vi "AeroQuadConfigurator.vi"() -> ()   [LabVIEW 2010]
uses:
  <vilib>/Utility/config.llb/Config Data RefNum.ctl
  <vilib>/Utility/miscctls.llb/LVRowAndColumnTypeDef.ctl
  <vilib>/Utility/miscctls.llb/LVRowAndColumnUnsignedTypeDef.ctl
  <vilib>/Utility/config.llb/Read Key (Double).vi
  <vilib>/Utility/config.llb/Read Key (String).vi
  <vilib>/Utility/config.llb/Read Key (I32).vi
  <vilib>/Utility/config.llb/Write Key (I32).vi
  <vilib>/Utility/config.llb/Write Key (String).vi
  <vilib>/Platform/browser.llb/Open URL in Default Browser (string).vi
  <vilib>/Instr/_visa.llb/VISA Configure Serial Port (Instr).vi
  <vilib>/Utility/config.llb/NI_LVConfig.lvlib
panel:
  out "LargeStatus":string
  in  "Load SubPanel":i32(ring) caption="Information Display" items=["Initial Setup", "3-D View", "Vehicle Status", "Map Tracker", "Motor Commands", "Serial Monitor", "Vehicle Attitude", "Sensor Data", "Transmitter Data"]
  in  "Parameter Type":i32(ring) caption="Configuration" items=["Rate Mode", "Attitude Mode", "Yaw Configuration", "Altitude Hold", "Miscellaneous Configuration", "Transmitter Smoothing", "Battery Monitor", "Camera Stabilization"]
  in  "Parameter Check":string[][](table)
  in  "Upload":bool
  out "Sensors":string[][](table)
  out "Status":string="AeroQuad Configurator"
  in  "*Com Port":refnum<visa-resource-name> caption="Com Port"
  in  "*Baud Rate":string(combo)="115200" caption="Baud Rate"
  in  "*Timeout (sec)":dbl=3.0 caption="Timeout (sec)"
  in  "Open Port":bool
  in  "Disconnect":bool
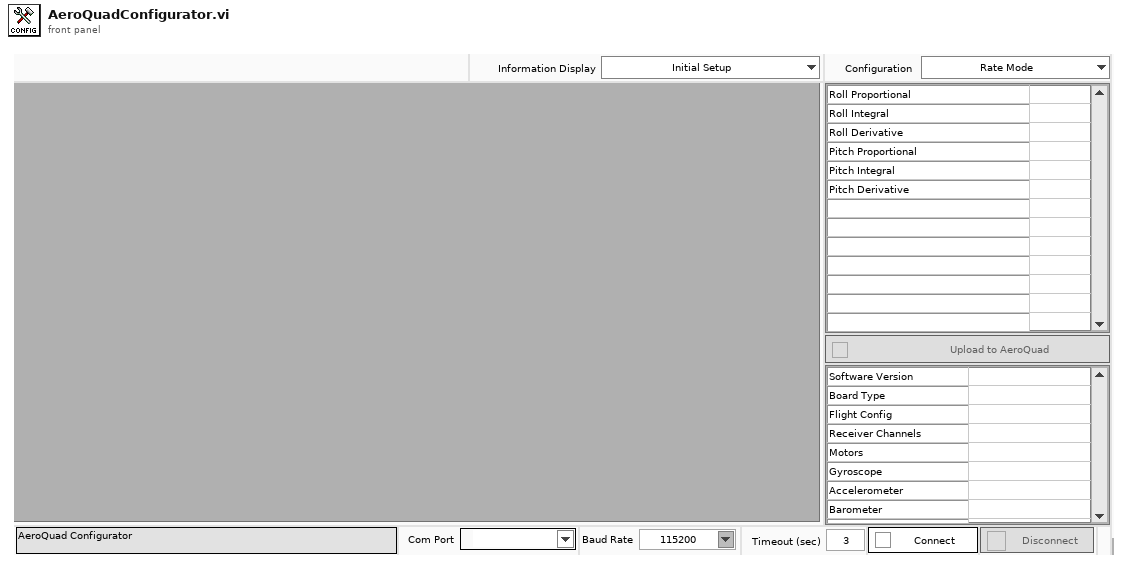
[diagram p1: front panel]
types:
  T1 = typedef "NI_LVConfig.lvlib/Config Data RefNum.ctl" = refnum<k1>
  T2 = cluster{"Error":errorcluster, "Data":dbl[], "COM Port":refnum<visa-resource-name>, "Data Type":enum16{"Serial", "Binary"}, "Connected":bool, "Parameters":string[][][], "WorkingPath":path, "ConfigRef":T1, "SubPanelName":string[], "ParameterName":string[], "Plots":string[][][], "SubPanelQueue":refnum<queue>, "SubPanel":refnum<vi>, "Debug":bool, "SubPanelType":string[], "Version":string, "StopTelem":string, "Config":string[][], "oldTelem":string, "previousValid":string, "oldCmd":string, "StartDelay":dbl, "ParamDesc":string[][], "IniPath":path, "SW":string}
  T3 = enum8{"Enabled", "Disabled", "Disabled and Grayed Out"}
  T4 = cluster{"Section":string, "Key":string, "Value":string}
  T5 = typedef "LVRowAndColumnTypeDef.ctl" = cluster{"Row":i32, "Column":i32}
  T6 = typedef "LVRowAndColumnUnsignedTypeDef.ctl" = cluster{"Row":u32, "Column":u32}
  T7 = enum32{"invalid app kind", "Development System", "Run Time System", "Student Edition", "Embedded LabVIEW", "Evaluation", "Custom"}
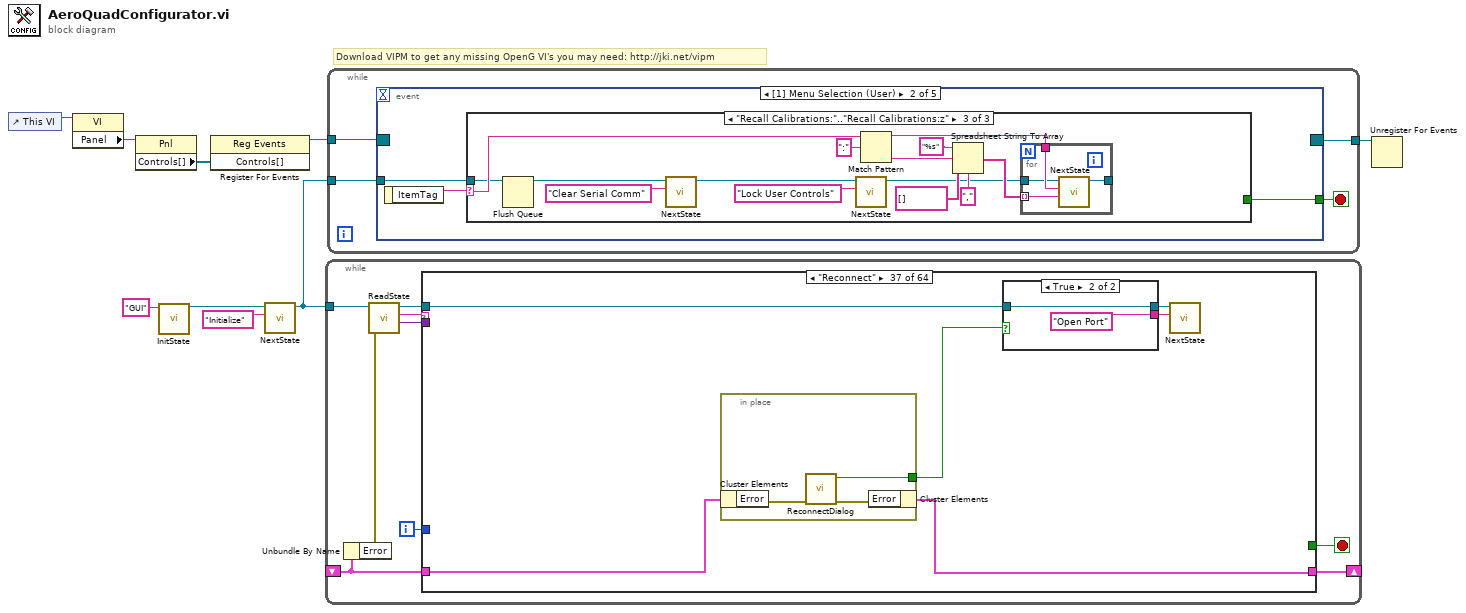
[diagram p0: block diagram]
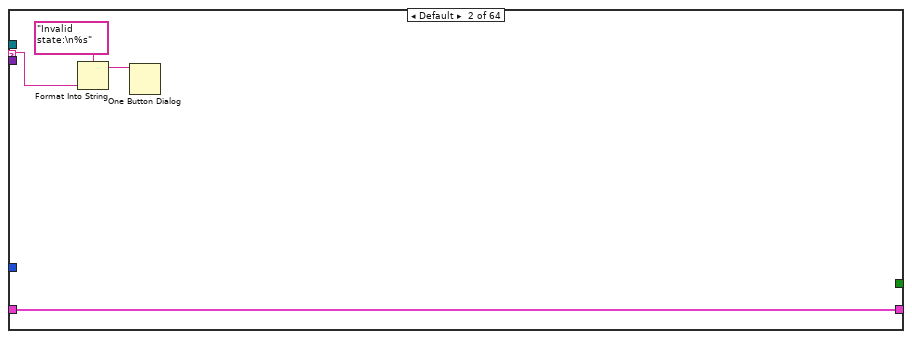
[diagram p3: hidden frame]
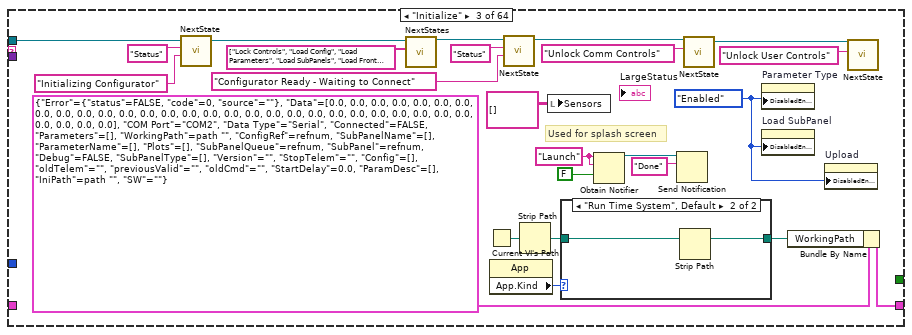
[diagram p4: hidden frame]
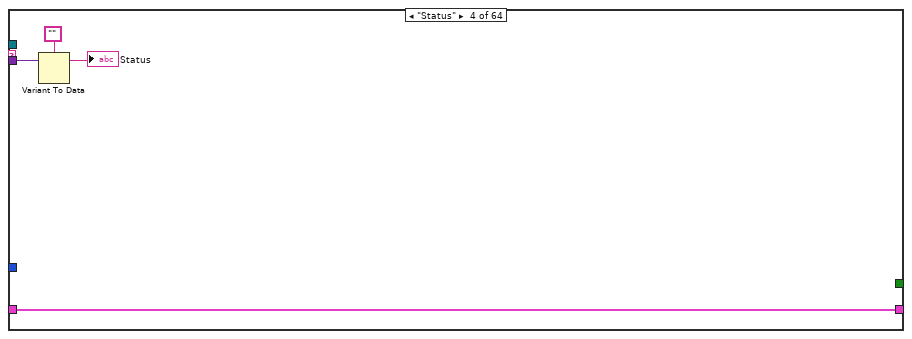
[diagram p6: hidden frame]
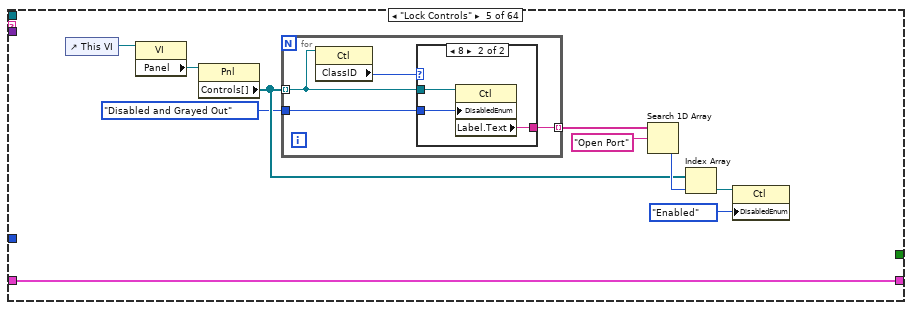
[diagram p7: hidden frame]
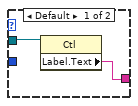
[diagram p8: hidden frame]
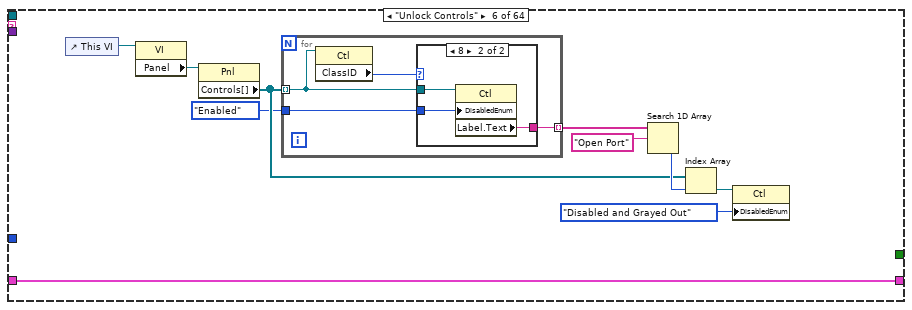
[diagram p9: hidden frame]
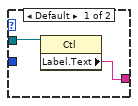
[diagram p10: hidden frame]
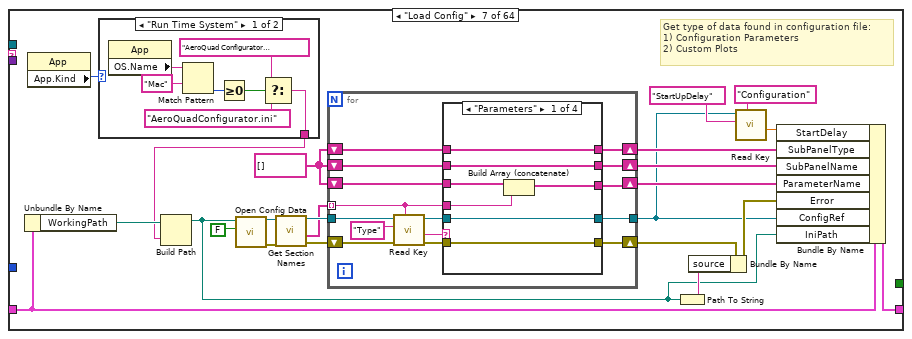
[diagram p11: hidden frame]
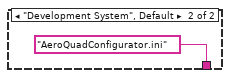
[diagram p12: hidden frame]
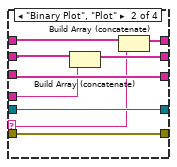
[diagram p13: hidden frame]
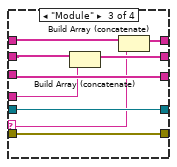
[diagram p14: hidden frame]
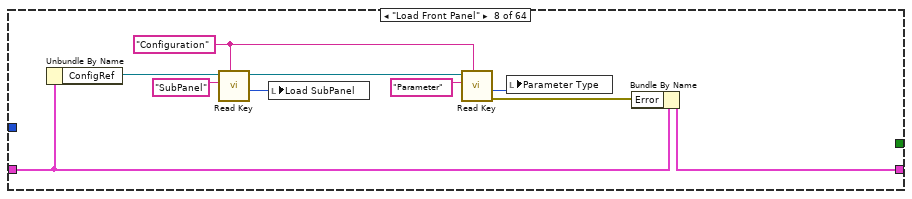
[diagram p16: hidden frame]
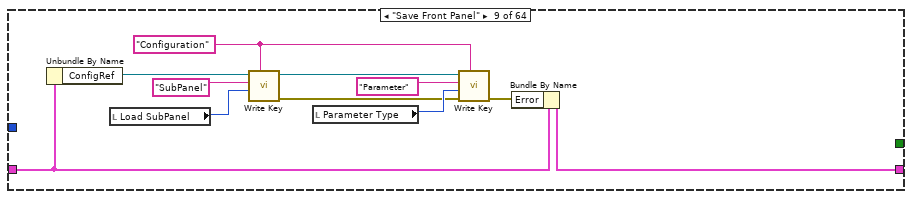
[diagram p17: hidden frame]
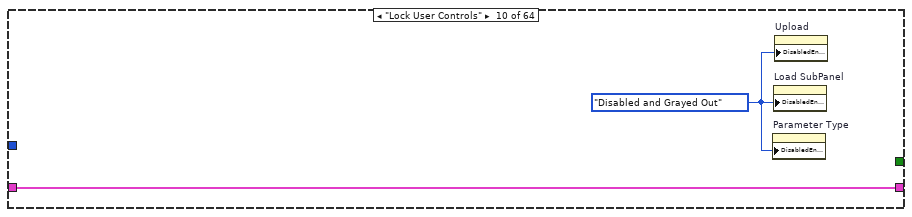
[diagram p18: hidden frame]
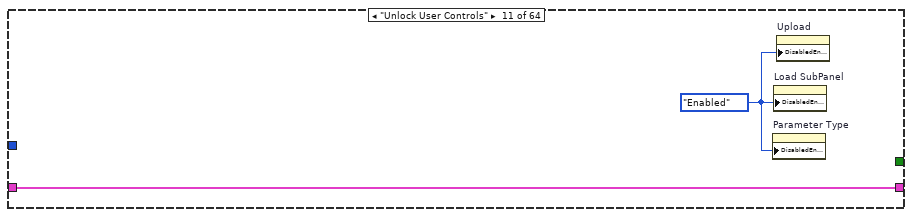
[diagram p19: hidden frame]
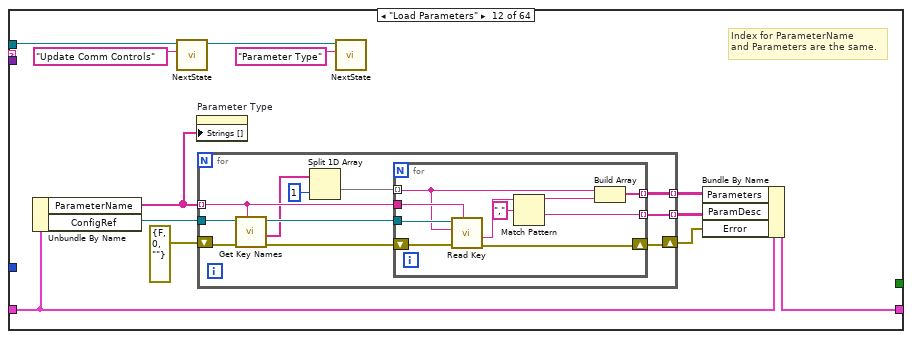
[diagram p20: hidden frame]
diagram:
  # "Download VIPM to get any missing OpenG VI's you may need: http://jki.net/vipm"
  n1 = control-ref of="This VI"() -> (w9:refnum<vi>)
  n2 = property class="VI"(reference=w9) -> ("Panel"=w8:refnum<vi>)  [unwired: 1 in, 2 out]
  n3 = property class="Pnl"(reference=w8) -> ("Controls[]"=w7:refnum<vi>[])  [unwired: 1 in, 2 out]
  n4 = call "InitState.vi"("Name"="GUI") -> ("Queue Out"=w2:refnum<queue>)  [unwired: 8 in, 1 out]
  n5 = register-events(w7) -> (reference out=w6:refnum<event-registration>)  [unwired: 2 in, 1 out]
  n6 = call "NextState.vi"("State"="Initialize", "Queue In"=w2) -> ("Queue Out"=w3:refnum<queue>)  [unwired: 8 in, 1 out]
  n7 = while {
    tunnel: w3 -> [w13]
    shift-right: [w18] -> _
    shift-left: _ -> [w15]
    i -> [w16]
    stop <- w17 stop-if-true
    n8 = Unbundle By Name(w15) -> ("Error"=w14:errorcluster)
    n9 = call "ReadState.vi"("Error In"=w14, "Queue In"=w13) -> ("Data"=w10:variant, "State"=w11:string, "Queue Out"=w12:refnum<queue>)  [unwired: 6 in, 1 out]
    n10 = case shown="\"Reconnect\"" w11 {
      tunnel: w10 -> [_ _ _ w51 _ _ _ _ _ _ _ _ _ w248 w263 _ _ _ w320 w326 _ _ _ _ _ _ _ _ _ w482 w486 _ _ _ w623 _ _ _ w689 _ _ _ _ _ _ _ w892 _ _ _ _ _ _ w993 _ _ _ w1117 w1132 _ _ w1241 w1253 w1321]
      selector: w11 -> [_ w22 _ _ _ _ _ _ _ _ _ _ _ _ w253 _ _ _ _ _ _ _ _ _ _ _ _ _ _ _ _ _ _ _ w619 _ _ _ _ _ _ _ _ _ _ _ _ _ _ _ _ _ _ _ _ _ _ _ _ _ _ w1240 w1252 _]
      tunnel: [w19 w23 w36 w52 w56 w75 w111 w171 w187 w191 w193 w204 w237 w250 w264 w282 w314 w317 w321 w327 w329 w339 w342 w377 w432 w433 w462 w474 w476 w481 w487 w506 w540 w596 w624 w640 w664 w684 w686 w695 w697 w711 w743 w758 w820 w881 w890 w905 w906 w910 w931 w948 w967 w995 w1044 w1050 w1052 w1120 w1180 w1186 w1223 w1236 w1250 w1327] -> w18
      tunnel: [_ _ _ _ _ _ _ _ _ _ _ _ _ _ _ _ _ _ _ _ _ TRUE _ _ _ _ _ _ _ _ _ _ _ _ _ _ _ _ _ _ _ _ _ _ _ _ _ _ _ _ _ _ _ _ _ _ _ _ _ _ _ _ _ _] -> w17
      tunnel: w15 -> [w19 w23 _ w52 w56 w75 w112 w172 w188 w191 w193 w205 w238 w251 w264 w283 w314 w317 w321 w327 w329 w339 w342 w378 w432 w434 w462 w474 w476 w481 w487 w492 w541 w597 w625 w641 w665 w685 w686 w695 w697 w711 w743 w759 w821 w881 w890 w905 w906 w911 w932 w949 w968 w996 w1044 w1050 w1053 w1120 w1180 w1186 w1223 w1237 w1250 w1327]
      tunnel: w16 -> [_ _ _ _ _ _ _ _ _ _ _ _ _ _ _ w284 _ _ _ _ _ _ _ _ _ _ _ _ _ _ _ _ _ _ _ _ _ _ _ _ _ _ _ _ _ _ _ _ _ _ _ _ _ _ _ _ _ _ _ _ _ _ _ _]
      tunnel: w12 -> [_ _ w47 _ _ _ _ _ _ _ _ w198 w228 _ w257 w280 _ w316 _ _ _ w340 _ w351 _ _ _ _ _ _ w483 w497 w543 w595 w620 _ w663 w681 _ _ _ _ _ _ _ w835 _ w894 _ w908 w929 _ w964 w990 w1038 _ w1054 w1115 w1145 _ _ _ w1247 w1326]
      frame "--- System ---" {
      }
      frame Default {
        n11 = Format Into String(format string="Invalid state:\n%s", w22) -> (resulting string=w20:string)  [unwired: 2 in, 1 out]
        n12 = One Button Dialog(message=w20) -> ()  [unwired: 1 in, 1 out]
      }
      frame "Initialize" {
        w27 = "Launch" ("name (unnamed)")
        w28 = T3."Enabled" ("Disabled")
        # "Used for splash screen"
        n13 = call "NextState.vi"("Data"="Initializing Configurator", "State"="Status", "Queue In"=w47) -> ("Queue Out"=w30:refnum<queue>)  [unwired: 7 in, 1 out]
        n14 = call "NextStates.vi"("States"=string[] ["Lock Controls", "Load Config", "Load Parameters", "Load SubPanels", "Load Front Panel"], "Queue In"=w30) -> ("Queue Out"=w29:refnum<queue>)  [unwired: 8 in, 1 out]
        n15 = Current VI's Path() -> (path=w39:path)
        n16 = property class="App"() -> ("App.Kind"=w41:T7)  [unwired: 2 in, 2 out]
        n17 = call "NextState.vi"("Data"="Configurator Ready - Waiting to Connect", "State"="Status", "Queue In"=w29) -> ("Queue Out"=w35:refnum<queue>)  [unwired: 7 in, 1 out]
        n18 = Strip Path(path=w39) -> (stripped path=w40:path)  [unwired: 1 out]
        n19 = local write "Sensors"(string[][] [] ("Sensors")) -> ()
        n20 = case shown="\"Run Time System\", Default" w41 {
          tunnel: w40 -> [w48 w50]
          tunnel: [w48 w49] -> w38
          frame "Development System" {
          }
          frame "Run Time System", Default {
            n21 = Strip Path(path=w50) -> (stripped path=w49:path)  [unwired: 1 out]
          }
        }
        n22 = Obtain Notifier(name (unnamed)=w27, notification data type=w27, create if not found? (T)=FALSE) -> (notifier out=w25:refnum<notifier>)  [unwired: 1 in, 2 out]
        n23 = Send Notification(notification="Done", notifier=w25) -> ()  [unwired: 1 in, 2 out]
        n24 = call "NextState.vi"("State"="Unlock Comm Controls", "Queue In"=w35) -> ("Queue Out"=w33:refnum<queue>)  [unwired: 8 in, 1 out]
        n25 = property on="Parameter Type" class="Ring (strict)"("DisabledEnum"=w28) -> ()  [unwired: 2 in, 2 out]
        n26 = property on="Load SubPanel" class="Ring (strict)"("DisabledEnum"=w28) -> ()  [unwired: 2 in, 2 out]
        n27 = Bundle By Name(cluster=T2 {"Error"={"status"=FALSE, "code"=0, "source"=""}, "Data"=[0.0, 0.0, 0.0, 0.0, 0.0, 0.0, 0.0, 0.0, 0.0, 0.0, 0.0, 0.0, 0.0, 0.0, 0.0, 0.0, 0.0, 0.0, 0.0, 0.0, 0.0, 0.0, 0.0, 0.0, 0.0, 0.0, 0.0, 0.0, 0.0, 0.0, 0.0, 0.0], "COM Port"="COM2", "Data Type"=enum."Serial", "Connected"=FALSE, "Parameters"=[], "WorkingPath"=path "", "ConfigRef"=refnum, "SubPanelName"=[], "ParameterName"=[], "Plots"=[], "SubPanelQueue"=refnum, "SubPanel"=refnum, "Debug"=FALSE, "SubPanelType"=[], "Version"="", "StopTelem"="", "Config"=[], "oldTelem"="", "previousValid"="", "oldCmd"="", "StartDelay"=0.0, "ParamDesc"=[], "IniPath"=path "", "SW"=""}, "WorkingPath"=w38) -> (w36:T2)
        n28 = property on="Upload" class="Bool"("DisabledEnum"=w28) -> ()  [unwired: 2 in, 2 out]
        n29 = call "NextState.vi"("State"="Unlock User Controls", "Queue In"=w33) -> ()  [unwired: 8 in, 2 out]
      }
      frame "Status" {
        n30 = Variant To Data(Variant=w51, type="") -> (data=→"Status":string)  [unwired: 1 in, 1 out]
      }
      frame "Lock Controls" {
        n31 = control-ref of="This VI"() -> (w63:refnum<vi>)
        n32 = property class="VI"(reference=w63) -> ("Panel"=w64:refnum<vi>)  [unwired: 1 in, 2 out]
        n33 = property class="Pnl"(reference=w64) -> ("Controls[]"=w59:refnum<vi>[])  [unwired: 1 in, 2 out]
        n34 = for {
          tunnel: w59 -> [w67] mode=indexing
          tunnel: [w68] -> w62 mode=indexing
          tunnel: T3."Disabled and Grayed Out" ("Disabled") -> [w65]
          n35 = property class="Ctl"(reference=w67) -> ("ClassID"=w66:u32)  [unwired: 1 in, 2 out]
          n36 = case shown="8" w66 {
            tunnel: [w69 w73] -> w68
            tunnel: w67 -> [w70 w72]
            tunnel: w65 -> [_ w71]
            frame Default {
              n37 = property class="Ctl"(reference=w70) -> ("Label.Text"=w69:string)  [unwired: 1 in, 2 out]
            }
            frame 8 {
              n38 = property class="Ctl"(reference=w72, "DisabledEnum"=w71) -> ("Label.Text"=w73:string)  [unwired: 1 in, 2 out]
            }
          }
        }
        n39 = Search 1D Array(1D array=w62, element="Open Port") -> (index of element=w60:i32)  [unwired: 1 in]
        n40 = Index Array(array=w59, index=w60) -> (element=w58:refnum<vi>)
        n41 = property class="Ctl"(reference=w58, "DisabledEnum"=T3."Enabled" ("Disabled")) -> ()  [unwired: 1 in, 2 out]
      }
      frame "Unlock Controls" {
        n42 = control-ref of="This VI"() -> (w82:refnum<vi>)
        n43 = property class="VI"(reference=w82) -> ("Panel"=w83:refnum<vi>)  [unwired: 1 in, 2 out]
        n44 = property class="Pnl"(reference=w83) -> ("Controls[]"=w78:refnum<vi>[])  [unwired: 1 in, 2 out]
        n45 = for {
          tunnel: w78 -> [w86] mode=indexing
          tunnel: [w87] -> w81 mode=indexing
          tunnel: T3."Enabled" ("Disabled") -> [w84]
          n46 = property class="Ctl"(reference=w86) -> ("ClassID"=w85:u32)  [unwired: 1 in, 2 out]
          n47 = case shown="8" w85 {
            tunnel: [w88 w92] -> w87
            tunnel: w86 -> [w89 w91]
            tunnel: w84 -> [_ w90]
            frame Default {
              n48 = property class="Ctl"(reference=w89) -> ("Label.Text"=w88:string)  [unwired: 1 in, 2 out]
            }
            frame 8 {
              n49 = property class="Ctl"(reference=w91, "DisabledEnum"=w90) -> ("Label.Text"=w92:string)  [unwired: 1 in, 2 out]
            }
          }
        }
        n50 = Search 1D Array(1D array=w81, element="Open Port") -> (index of element=w79:i32)  [unwired: 1 in]
        n51 = Index Array(array=w78, index=w79) -> (element=w77:refnum<vi>)
        n52 = property class="Ctl"(reference=w77, "DisabledEnum"=T3."Disabled and Grayed Out" ("Disabled")) -> ()  [unwired: 1 in, 2 out]
      }
      frame "Load Config" {
        w98 = string[] []
        # "Get type of data found in configuration file:\n1) Configuration Parameters\n2) Custom Plots"
        n53 = Unbundle By Name(w112) -> ("WorkingPath"=w110:path)
        n54 = property class="App"() -> ("App.Kind"=w100:T7)  [unwired: 2 in, 2 out]
        n55 = case shown="\"Run Time System\"" w100 {
          tunnel: [w116 "AeroQuadConfigurator.ini" ("name or relative path")] -> w101
          frame "Run Time System" {
            n56 = property class="App"() -> ("OS.Name"=w122:string)  [unwired: 2 in, 2 out]
            n57 = Match Pattern(string=w122, regular expression="Mac") -> (offset past match=w120:i32)  [unwired: 1 in, 3 out]
            n58 = Greater Or Equal To 0?(x=w120) -> (x >= 0?=w119:bool)
            n59 = Select(t="AeroQuad Configurator preferences" ("name or relative path"), s=w119, f="AeroQuadConfigurator.ini" ("name or relative path")) -> (s? t:f=w116:string)
          }
          frame "Development System", Default {
          }
        }
        n60 = Build Path(base path=w110, name or relative path=w101) -> (appended path=w93:path)
        n61 = call <vilib>:"Open Config Data.vi"("create file if necessary (T)"=FALSE, "configuration file path"=w93) -> ("error out"=w113:errorcluster, "refnum"=w114:T1)  [unwired: 7 in, 1 out]
        n62 = call <vilib>:"Get Section Names.vi"("error in (no error)"=w113, "refnum"=w114) -> ("error out"=w107:errorcluster, "section names"=w108:string[], "refnum out"=w109:T1)  [unwired: 7 in]
        n63 = for {
          tunnel: w109 -> [w138]
          tunnel: w108 -> [w127] mode=indexing
          shift-right: [w134] -> w104
          shift-left: w107 -> [w136]
          tunnel: [w132] -> w94
          shift-right: [w131] -> w106
          shift-left: w98 -> [w130]
          shift-right: [w128] -> w105
          shift-left: w98 -> [w129]
          shift-right: [w124] -> w99
          shift-left: w98 -> [w125]
          n64 = call-poly <vilib>:"Read Key.vi"("section"=w127, "error in (no error)"=w136, "key"="Type", "refnum"=w138) -> ("error out"=w135:errorcluster, "value"=w126:string, "refnum out"=w133:T1)  [unwired: 4 in, 1 out]
          n65 = case shown="\"Parameters\"" w126 {
            selector: w126 -> [_ w147 w156 _]
            tunnel: [w142 w153 w162 w168] -> w134
            tunnel: w135 -> [w142 w153 w162 w168]
            tunnel: [w143 w154 w163 w167] -> w132
            tunnel: w133 -> [w143 w154 w163 w167]
            tunnel: [w145 w150 w159 w166] -> w131
            tunnel: w130 -> [w144 w150 w159 w166]
            tunnel: [w141 w151 w160 w165] -> w128
            tunnel: w129 -> [w141 w152 w161 w165]
            tunnel: w127 -> [w140 w149 w158 _]
            tunnel: w125 -> [w139 w148 w157 w164]
            tunnel: [w139 w146 w155 w164] -> w124
            frame "Parameters" {
              n66 = Build Array (concatenate)(w144, w140) -> (w145:string[])
            }
            frame "Binary Plot", "Plot" {
              n67 = Build Array (concatenate)(w152, w149) -> (w151:string[])
              n68 = Build Array (concatenate)(w148, w147) -> (w146:string[])
            }
            frame "Module" {
              n69 = Build Array (concatenate)(w161, w158) -> (w160:string[])
              n70 = Build Array (concatenate)(w157, w156) -> (w155:string[])
            }
            frame Default {
            }
          }
        }
        n71 = Path To String(path=w93) -> (string=w102:string)
        n72 = Bundle By Name(cluster=w104, "source"=w102) -> (w103:errorcluster)
        n73 = call-poly <vilib>:"Read Key.vi"("section"="Configuration", "key"="StartUpDelay", "refnum"=w94) -> ("value"=w95:dbl)  [unwired: 5 in, 3 out]
        n74 = Bundle By Name(cluster=w112, "StartDelay"=w95, "SubPanelType"=w99, "SubPanelName"=w105, "ParameterName"=w106, "Error"=w103, "ConfigRef"=w94, "IniPath"=w93) -> (w111:T2)
      }
      frame "Load Front Panel" {
        w169 = "Configuration" ("section")
        n75 = Unbundle By Name(w172) -> ("ConfigRef"=w178:T1)
        n76 = call-poly <vilib>:"Read Key.vi"("section"=w169, "key"="SubPanel", "refnum"=w178) -> ("value"=w176:i32, "refnum out"=w174:T1)  [unwired: 5 in, 2 out]
        n77 = local write "Load SubPanel"(w176) -> ()
        n78 = call-poly <vilib>:"Read Key.vi"("section"=w169, "key"="Parameter", "refnum"=w174) -> ("error out"=w170:errorcluster, "value"=w173:i32)  [unwired: 5 in, 2 out]
        n79 = local write "Parameter Type"(w173) -> ()
        n80 = Bundle By Name(cluster=w172, "Error"=w170) -> (w171:T2)
      }
      frame "Save Front Panel" {
        w182 = "Configuration" ("section")
        n81 = Unbundle By Name(w188) -> ("ConfigRef"=w189:T1)
        n82 = local read "Load SubPanel"() -> (w185:i32)
        n83 = call-poly <vilib>:"Write Key.vi"("section"=w182, "value"=w185, "key"="SubPanel", "refnum"=w189) -> ("error out"=w180:errorcluster, "refnum out"=w183:T1)  [unwired: 5 in, 1 out]
        n84 = local read "Parameter Type"() -> (w181:i32)
        n85 = call-poly <vilib>:"Write Key.vi"("section"=w182, "error in (no error)"=w180, "value"=w181, "key"="Parameter", "refnum"=w183) -> ("error out"=w179:errorcluster)  [unwired: 4 in, 2 out]
        n86 = Bundle By Name(cluster=w188, "Error"=w179) -> (w187:T2)
      }
      frame "Lock User Controls" {
        w190 = T3."Disabled and Grayed Out" ("Disabled")
        n87 = property on="Parameter Type" class="Ring (strict)"("DisabledEnum"=w190) -> ()  [unwired: 2 in, 2 out]
        n88 = property on="Load SubPanel" class="Ring (strict)"("DisabledEnum"=w190) -> ()  [unwired: 2 in, 2 out]
        n89 = property on="Upload" class="Bool"("DisabledEnum"=w190) -> ()  [unwired: 2 in, 2 out]
      }
      frame "Unlock User Controls" {
        w192 = T3."Enabled" ("Disabled")
        n90 = property on="Parameter Type" class="Ring (strict)"("DisabledEnum"=w192) -> ()  [unwired: 2 in, 2 out]
        n91 = property on="Load SubPanel" class="Ring (strict)"("DisabledEnum"=w192) -> ()  [unwired: 2 in, 2 out]
        n92 = property on="Upload" class="Bool"("DisabledEnum"=w192) -> ()  [unwired: 2 in, 2 out]
      }
      frame "Load Parameters" {
        # "Index for ParameterName\nand Parameters are the same."
        n93 = Unbundle By Name(w205) -> ("ParameterName"=w199:string[], "ConfigRef"=w202:T1)
        n94 = call "NextState.vi"("State"="Update Comm Controls", "Queue In"=w198) -> ("Queue Out"=w197:refnum<queue>)  [unwired: 8 in, 1 out]
        n95 = property on="Parameter Type" class="Ring (strict)"("Strings []"=w199) -> ()  [unwired: 2 in, 2 out]
        n96 = for {
          shift-right: [w210] -> w195
          shift-left: errorcluster {"status"=FALSE, "code"=0, "source"=""} ("error out") -> [w216]
          tunnel: w202 -> [w215]
          tunnel: w199 -> [w212] mode=indexing
          tunnel: [w211] -> w200 mode=indexing
          tunnel: [w206] -> w194 mode=indexing
          n97 = call <vilib>:"Get Key Names.vi"("section"=w212, "error in (no error)"=w216, "refnum"=w215) -> ("error out"=w214:errorcluster, "key names"=w209:string[], "refnum out"=w213:T1)  [unwired: 5 in, 1 out]
          n98 = Split 1D Array(array=w209, index=1) -> (second subarray=w207:string[])  [unwired: 1 out]
          n99 = for {
            shift-right: [w222] -> w210
            shift-left: w214 -> [w226]
            tunnel: w213 -> [w225]
            tunnel: w207 -> [w223] mode=indexing
            tunnel: w212 -> [w224]
            tunnel: [w221] -> w211 mode=indexing
            tunnel: [w217] -> w206 mode=indexing
            n100 = call-poly <vilib>:"Read Key.vi"("section"=w224, "error in (no error)"=w226, "key"=w223, "refnum"=w225) -> ("error out"=w222:errorcluster, "value"=w220:string)  [unwired: 4 in, 2 out]
            n101 = Match Pattern(string=w220, regular expression=",") -> (before substring=w218:string, after substring=w217:string)  [unwired: 1 in, 2 out]
            n102 = Build Array(w223, w218) -> (w221:string[])
          }
        }
        n103 = call "NextState.vi"("State"="Parameter Type", "Queue In"=w197) -> ()  [unwired: 8 in, 2 out]
        n104 = Bundle By Name(cluster=w205, "Parameters"=w200, "ParamDesc"=w194, "Error"=w195) -> (w204:T2)
      }
      frame "Load SubPanels" {
        # "Load SubPanel names, add custom plots at end."
        n105 = call "NextState.vi"("State"="Load SubPanel", "Queue In"=w228) -> ()  [unwired: 8 in, 2 out]
        n106 = Unbundle By Name(w238) -> ("SubPanelName"=w227:string[], "ConfigRef"=w231:T1)
        n107 = for {
          tunnel: w231 -> [w242]
          tunnel: [w241] -> w230 mode=indexing
          tunnel: w227 -> [w239] mode=indexing
          tunnel: [w240] -> w229 mode=indexing
          n108 = call "GetSectionData.vi"("SectionName"=w239, "ConfigRef"=w242) -> ("error out"=w241:errorcluster, "Data"=w240:string[][])  [unwired: 7 in, 1 out]
        }
        n109 = property on="Load SubPanel" class="Ring (strict)"("Strings []"=w227) -> ()  [unwired: 2 in, 2 out]
        n110 = Merge Errors(w230) -> (w236:errorcluster)
        n111 = Obtain Queue(name (unnamed)="SubPanel", element data type=cluster{"State":string, "Data":variant} {"State"="", "Data"=variant}) -> (queue out=w232:refnum<queue>)  [unwired: 3 in, 2 out]
        n112 = Bundle By Name(cluster=w238, "Plots"=w229, "Error"=w236, "SubPanelQueue"=w232) -> (w237:T2)
      }
      frame "Save Configuration" {
        n113 = Variant To Data(Variant=w248, type=T4 {"Section"="", "Key"="", "Value"=""}) -> (data=w246:T4)  [unwired: 1 in, 1 out]
        n114 = Unbundle By Name(w246) -> ("Section"=w245:string, "Key"=w244:string, "Value"=w243:string)
        n115 = Unbundle By Name(w251) -> ("ConfigRef"=w252:T1)
        n116 = call-poly <vilib>:"Write Key.vi"("section"=w245, "value"=w243, "key"=w244, "refnum"=w252) -> ("error out"=w249:errorcluster)  [unwired: 5 in, 2 out]
        n117 = Bundle By Name(cluster=w251, "Error"=w249) -> (w250:T2)
      }
      frame "Menu Link" {
        w262 = "199.193.247.52"  # www.AeroQuad.com
        n118 = Variant To Data(Variant=w263, type=w253) -> (data=w254:string)  [unwired: 1 in, 1 out]
        n119 = case shown="\"Bug Reporting\"" w254 {
          tunnel: ["https://aeroquad.atlassian.net" ("URL") "http://aeroquad.com/showwiki.php?title=AeroQuad+3+x+Configurator+Manual" ("URL") "http://aeroquad.com/showwiki.php" ("URL") "http://aeroquad.com/forum.php" ("URL")] -> w255
          frame "Bug Reporting" {
          }
          frame "User Manual" {
          }
          frame "Documentation" {
          }
          frame "Forum", Default {
          }
        }
        n120 = TCP Open Connection(address=w262, remote port or service name=u16 80, timeout ms (60000)=3000) -> (connection ID=w258:refnum<k5>, error out=w259:errorcluster)  [unwired: 2 in]
        n121 = TCP Close Connection(connection ID=w258, error in (no error)=w259) -> (error out=w256:errorcluster)  [unwired: 1 in, 1 out]
        n122 = case shown="Error" w256 {
          tunnel: w257 -> [_ w268]
          tunnel: w255 -> [w265 _]
          tunnel: w254 -> [_ w267]
          tunnel: w253 -> [_ w266]
          frame No Error {
            n123 = call-poly <vilib>:"Open URL in Default Browser.vi"("URL"=w265) -> ()  [unwired: 5 in, 2 out]
          }
          frame Error {
            n124 = Two Button Dialog(message="This feature requires a network connection.", 2:"Retry" ("T button name (\"OK\")")) -> (T button?=w269:bool)  [unwired: 1 in]
            n125 = case shown="False" w269 {
              tunnel: w268 -> [_ w274]
              tunnel: w266 -> [_ w273]
              tunnel: w267 -> [_ w272]
              frame False {
              }
              frame True {
                n126 = call "NextState.vi"("Data"=w272, "State"=w273, "Queue In"=w274) -> ()  [unwired: 7 in, 2 out]
              }
            }
          }
        }
      }
      frame "Error" {
        n127 = Flush Queue(queue=w280) -> (queue out=w281:refnum<queue>)  [unwired: 1 in, 2 out]
        n128 = case shown="Default" w284 {
          tunnel: w283 -> [w286 w290]
          tunnel: [w285 w292] -> w282
          tunnel: w281 -> [_ w291]
          frame 0 {
            n129 = in-place {
              n130 = in-place-cluster #1(w286) -> ("Error"=w288:errorcluster)
              n131 = call <vilib>:"Clear Errors.vi"("error in (no error)"=w288) -> ("error out"=w287:errorcluster)  [unwired: 6 in]
              n132 = in-place-cluster #1("Error"=w287) -> (w285:T2)
            }
          }
          frame Default {
            n133 = Unbundle By Name(w290) -> ("Error.code"=w289:i32)
            n134 = case shown="7, 1003" w289 {
              tunnel: w290 -> [w298 w306]
              tunnel: [w297 w305] -> w292
              tunnel: w291 -> [w294 w304]
              frame 7, 1003 {
                n135 = Unbundle By Name(w298) -> ("Error"=w299:errorcluster)
                n136 = call "NextState.vi"("State"="Load SubPanel", "Queue In"=w294) -> ()  [unwired: 8 in, 2 out]
                n137 = call <vilib>:"Clear Errors.vi"("error in (no error)"=w299) -> ("error out"=w296:errorcluster)  [unwired: 6 in]
                n138 = Bundle By Name(cluster=w298, "Error"=w296) -> (w297:T2)
                n139 = local write "Load SubPanel"(0) -> ()
                n140 = One Button Dialog(message="This feature is currently not supported in this version of the Configurator") -> ()  [unwired: 1 in, 1 out]
              }
              frame Default {
                n141 = in-place {
                  in-place-border: [w310] -> w301
                  n142 = in-place-cluster #2(w306) -> ("Connected"=w310:bool, "Error"=w312:errorcluster)
                  n143 = call "ErrorDialog.vi"("error in"=w312) -> ("error out"=w311:errorcluster)  [unwired: 10 in]
                  n144 = call <vilib>:"Clear Errors.vi"("error in (no error)"=w311) -> ("error out"=w313:errorcluster)  [unwired: 6 in]
                  n145 = in-place-cluster #2("Connected"=FALSE, "Error"=w313) -> (w305:T2)
                }
                n146 = call "NextState.vi"("State"="Disconnect", "Queue In"=w304) -> ("Queue Out"=w302:refnum<queue>)  [unwired: 8 in, 1 out]
                n147 = case shown="True" w301 {
                  tunnel: w302 -> [_ w308]
                  frame False {
                  }
                  frame True {
                    n148 = call "NextState.vi"("State"="Reconnect", "Queue In"=w308) -> ()  [unwired: 8 in, 2 out]
                  }
                }
              }
            }
          }
        }
        n149 = local write "Status"("Error detected!" ("Status")) -> ()
      }
      frame "About" {
        n150 = One Button Dialog(message="AeroQuad Configurator v3.1 Beta 1") -> ()  [unwired: 1 in, 1 out]
      }
      frame "Clear Queue" {
        n151 = Flush Queue(queue=w316) -> ()  [unwired: 1 in, 3 out]
      }
      frame "Delay" {
        n152 = Variant To Data(Variant=w320, type=u32 0 ("milliseconds to wait")) -> (data=w318:u32)  [unwired: 1 in, 1 out]
        n153 = Wait (ms)(milliseconds to wait=w318) -> ()  [unwired: 1 out]
      }
      frame "Delay String" {
        n154 = Variant To Data(Variant=w326, type="") -> (data=w324:string)  [unwired: 1 in, 1 out]
        n155 = Decimal String To Number(string=w324) -> (number=w323:i32)  [unwired: 2 in, 1 out]
        n156 = To Unsigned Long Integer(number=w323) -> (unsigned 32bit integer=w322:u32)
        n157 = Wait (ms)(milliseconds to wait=w322) -> ()  [unwired: 1 out]
      }
      frame "Delay SubPanel" {
        n158 = Wait (ms)(milliseconds to wait=u32 250) -> ()  [unwired: 1 out]
      }
      frame "Exit" {
        n159 = Unbundle By Name(w339) -> ("Debug"=w333:bool, "SubPanel"=w335:refnum<vi>, "SubPanelQueue"=w336:refnum<queue>, "ConfigRef"=w338:T1, "COM Port"=w332:refnum<visa-resource-name>, "StopTelem"=w330:string)
        n160 = Release Queue(queue=w340) -> ()  [unwired: 2 in, 3 out]
        n161 = VISA Write(VISA resource name=w332, write buffer=w330) -> (VISA resource name out=w331:refnum<visa-resource-name>)  [unwired: 1 in, 2 out]
        n162 = VISA Close(VISA resource name=w331) -> ()  [unwired: 1 in, 1 out]
        n163 = call <vilib>:"Close Config Data.vi"("write file if changed (T)"=TRUE, "refnum"=w338) -> ()  [unwired: 8 in, 2 out]
        n164 = Release Queue(queue=w336) -> ()  [unwired: 2 in, 3 out]
        n165 = invoke class="VI" method="Abort VI"(reference=w335) -> (reference out=w334:refnum<vi>)  [unwired: 2 in, 2 out]
        n166 = Close Reference(reference=w334) -> ()  [unwired: 1 in, 1 out]
        n167 = case shown="False" w333 {
          frame False {
            n168 = invoke class="VI" method="FP.Close"() -> ()  [unwired: 3 in, 3 out]
          }
          frame True {
          }
        }
      }
      frame "--- GUI ---" {
      }
      frame "Load SubPanel" {
        w343 = T3."Enabled" ("Disabled")
        # "Close previous panel."
        n169 = Unbundle By Name(w378) -> ("Config"=w344:string[][], "SubPanelType"=w349:string[], "ConfigRef"=w372:T1, "Plots"=w369:string[][][], "SubPanelName"=w347:string[], "WorkingPath"=w358:path, "SubPanelQueue"=w363:refnum<queue>, "COM Port"=w354:refnum<visa-resource-name>, "SubPanel"=w355:refnum<vi>)
        n170 = flat-sequence {
          tunnel: w355 -> [w383]
          tunnel: w354 -> [w382]
          tunnel: w351 -> [w380]
          tunnel: [w379] -> w353
          frame #0 {
            n171 = invoke class="VI" method="Abort VI"(reference=w383) -> (reference out=w384:refnum<vi>)  [unwired: 2 in, 2 out]
            n172 = Close Reference(reference=w384) -> ()  [unwired: 1 in, 1 out]
            n173 = VISA Write(VISA resource name=w382, write buffer="X") -> ()  [unwired: 1 in, 3 out]
            n174 = Flush Queue(queue=w380) -> (error out=w379:errorcluster)  [unwired: 1 in, 2 out]
          }
        }
        n175 = property on="Load SubPanel" class="Ring (strict)"() -> ("Strings []"=w373:string[])  [unwired: 2 in, 2 out]
        n176 = Index Array(array=w373, index="Load SubPanel") -> (element=w346:string)
        n177 = Search 1D Array(1D array=w347, element=w346) -> (index of element=w345:i32)  [unwired: 1 in]
        n178 = property class="App"() -> ("App.Kind"=w361:T7)  [unwired: 2 in, 2 out]
        n179 = Index Array(array=w349, index=w345) -> (element=w350:string)
        n180 = Flush Queue(queue=w363, error in (no error)=w353) -> (error out=w362:errorcluster)  [unwired: 2 out]
        n181 = case shown="\"Module\"" w350 {
          tunnel: w346 -> [_ w393 _ _]
          tunnel: w372 -> [_ w399 _ _]
          tunnel: w369 -> [_ _ w413 w426]
          tunnel: [_ w394 w412 w425] -> w368
          tunnel: [_ w395 _ _] -> w365
          tunnel: w361 -> [_ w392 w410 w423]
          tunnel: w358 -> [_ _ _ _]
          tunnel: [_ w391 w411 w424] -> w357
          tunnel: w345 -> [_ _ w409 w422]
          tunnel: w344 -> [_ w386 w408 w419]
          frame Default {
            n182 = One Button Dialog(message="Unknown module type. \nVerify INI file is correctly configured.") -> ()  [unwired: 1 in, 1 out]
          }
          frame "Module" {
            n183 = call-poly <vilib>:"Read Key.vi"("section"=w393, "key"="Path", "refnum"=w399) -> ("error out"=w397:errorcluster, "value"=w390:string, "refnum out"=w398:T1)  [unwired: 5 in, 1 out]
            n184 = call "GetSectionData.vi"("SectionName"=w393, "error in"=w397, "ConfigRef"=w398) -> ("error out"=w395:errorcluster, "Data"=w388:string[][])  [unwired: 6 in, 1 out]
            n185 = Build Array (concatenate)(w386, w388) -> (w387:string[][])
            n186 = call "FixMacPath.vi"("Input Path String"=w390) -> ("Output Path"=w389:path)  [unwired: 4 in]
            n187 = To Variant(anything=w387) -> (Variant=w394:variant)
            n188 = case shown="\"Development System\"" w392 {
              tunnel: [w401 w404] -> w391
              tunnel: w389 -> [w400 w405]
              frame "Run Time System", Default {
                n189 = Current VI's Path() -> (path=w403:path)
                n190 = Strip Path(path=w403) -> (stripped path=w402:path)  [unwired: 1 out]
                n191 = Build Path(base path=w402, name or relative path=w400) -> (appended path=w401:path)
              }
              frame "Development System" {
                n192 = call <userlib>:"Current VIs Parent Directory__ogtk.vi"("Relative path (.)"=w405) -> ("Parent Directory (+ Relative)"=w404:path)  [unwired: 4 in]
              }
            }
          }
          frame "Plot" {
            # "Custom Plot"
            n193 = Index Array(array=w413, index (dim 0)=w409) -> (element=w407:string[][])  [unwired: 2 in]
            n194 = Build Array (concatenate)(w408, w407) -> (w406:string[][])
            n195 = To Variant(anything=w406) -> (Variant=w412:variant)
            n196 = case shown="\"Run Time System\", Default" w410 {
              tunnel: [w416 path "Support/SubPanel/Plot/Plot.vi"] -> w411
              frame "Run Time System", Default {
                n197 = call "FixMacPath.vi"("Input Path String"="..\\Support\\SubPanel\\Plot\\Plot.vi" ("value")) -> ("Output Path"=w414:path)  [unwired: 4 in]
                n198 = Current VI's Path() -> (path=w417:path)
                n199 = Build Path(base path=w417, name or relative path=w414) -> (appended path=w416:path)
              }
              frame "Development System" {
              }
            }
          }
          frame "Binary Plot" {
            # "Custom Plot"
            n200 = Index Array(array=w426, index (dim 0)=w422) -> (element=w421:string[][])  [unwired: 2 in]
            n201 = Build Array (concatenate)(w419, w421) -> (w420:string[][])
            n202 = To Variant(anything=w420) -> (Variant=w425:variant)
            n203 = case shown="\"Run Time System\", Default" w423 {
              tunnel: [w429 path "Support/SubPanel/BinaryPlot/BinaryPlot.vi"] -> w424
              frame "Run Time System", Default {
                n204 = call "FixMacPath.vi"("Input Path String"="..\\Support\\SubPanel\\BinaryPlot\\BinaryPlot.vi" ("value")) -> ("Output Path"=w427:path)  [unwired: 4 in]
                n205 = Current VI's Path() -> (path=w430:path)
                n206 = Build Path(base path=w430, name or relative path=w427) -> (appended path=w429:path)
              }
              frame "Development System" {
              }
            }
          }
        }
        n207 = Open VI Reference(vi path=w357, error in (no error)=w362) -> (vi reference=w376:refnum<vi>, error out=w360:errorcluster)  [unwired: 4 in]
        n208 = Path To String(path=w357) -> (string=w356:string)
        n209 = Bundle By Name(cluster=w360, "source"=w356) -> (w359:errorcluster)
        n210 = invoke class="VI" method="Run VI"(reference=w376, error in=w359, "Wait until done"=FALSE ("Wait Until Done")) -> (reference out=w364:refnum<vi>, error out=w371:errorcluster)  [unwired: 2 in, 3 out]
        n211 = call "NextState.vi"("Error In"=w371, "Data"=w368, "State"="Initialize", "Queue In"=w363) -> ("Error Out"=w366:errorcluster)  [unwired: 6 in, 1 out]
        n212 = Merge Errors(w365, w366) -> (w367:errorcluster)
        n213 = invoke on="Sub Panel" class="SubPanel" method="Insert VI"(error in=w367, "VI Ref"=w364) -> (error out=w374:errorcluster)  [unwired: 2 in, 3 out]
        n214 = call "NextState.vi"("State"="Default Timeout", "Queue In"=w351) -> ()  [unwired: 8 in, 2 out]
        n215 = Bundle By Name(cluster=w378, "Error"=w374, "SubPanel"=w364) -> (w377:T2)
        n216 = property on="Parameter Type" class="Ring (strict)"("DisabledEnum"=w343) -> ()  [unwired: 2 in, 2 out]
        n217 = property on="Upload" class="Bool"("DisabledEnum"=w343) -> ()  [unwired: 2 in, 2 out]
      }
      frame "--- Communication ---" {
      }
      frame "Update Comm Controls" {
        w435 = "Configuration" ("section")
        # "In addition to comm controls,\nupdate commands/telemetry"
        n218 = Unbundle By Name(w434) -> ("ConfigRef"=w438:T1)
        n219 = call <vilib>:"Get Key Names.vi"("section"=w435, "refnum"=w438) -> ("key names"=w437:string[], "refnum out"=w436:T1)  [unwired: 6 in, 2 out]
        n220 = for {
          tunnel: w437 -> [w442] mode=indexing
          tunnel: w436 -> [w444]
          tunnel: w435 -> [w443]
          shift-right: [w439] -> w433
          shift-left: w434 -> [w440]
          n221 = call-poly <vilib>:"Read Key.vi"("section"=w443, "key"=w442, "refnum"=w444) -> ("value"=w441:string)  [unwired: 5 in, 3 out]
          n222 = case shown="\"SW\"" w442 {
            tunnel: w441 -> [_ w447 w449 w452 w453 w456 w459]
            tunnel: w440 -> [w445 w446 w448 w451 w454 w457 w461]
            tunnel: [w445 w446 w448 w451 w455 w458 w460] -> w439
            frame Default {
            }
            frame "COMport" {
              n223 = local write "*Com Port"(w447) -> ()
            }
            frame "Timeout" {
              n224 = Fract/Exp String To Number(string=w449) -> (number=w450:dbl)  [unwired: 3 in, 1 out]
              n225 = local write "*Timeout (sec)"(w450) -> ()
            }
            frame "Baud" {
              n226 = local write "*Baud Rate"(w452) -> ()
            }
            frame "Version" {
              n227 = Bundle By Name(cluster=w454, "Version"=w453) -> (w455:T2)
            }
            frame "StopTelem" {
              n228 = Bundle By Name(cluster=w457, "StopTelem"=w456) -> (w458:T2)
            }
            frame "SW" {
              n229 = Bundle By Name(cluster=w461, "SW"=w459) -> (w460:T2)
            }
          }
        }
      }
      frame "Save Comm Controls" {
        n230 = Unbundle By Name(w462) -> ("ConfigRef"=w464:T1)
        n231 = for {
          tunnel: string[] ["COMport", "Timeout", "Baud", ""] -> [w467] mode=indexing
          tunnel: w464 -> [w469]
          tunnel: "Configuration" ("section") -> [w468]
          n232 = case shown="\"Timeout\"" w467 {
            tunnel: [_ w470 w471 w473] -> w466
            frame Default {
            }
            frame "COMport" {
              n233 = local read "*Com Port"() -> (w470:refnum<visa-resource-name>)
            }
            frame "Timeout" {
              n234 = local read "*Timeout (sec)"() -> (w472:dbl)
              n235 = Number To Fractional String(number=w472) -> (F-format string=w471:string)  [unwired: 3 in]
            }
            frame "Baud" {
              n236 = local read "*Baud Rate"() -> (w473:string)
            }
          }
          n237 = call-poly <vilib>:"Write Key.vi"("section"=w468, "value"=w466, "key"=w467, "refnum"=w469) -> ()  [unwired: 5 in, 3 out]
        }
      }
      frame "Lock Comm Controls" {
        w475 = T3."Disabled and Grayed Out" ("Disabled")
        n238 = property on="*Com Port" class="VISAName"("DisabledEnum"=w475) -> ()  [unwired: 2 in, 2 out]
        n239 = property on="*Baud Rate" class="CmbBox"("DisabledEnum"=w475) -> ()  [unwired: 2 in, 2 out]
        n240 = property on="*Timeout (sec)" class="DigNum (strict)"("DisabledEnum"=w475) -> ()  [unwired: 2 in, 2 out]
      }
      frame "Unlock Comm Controls" {
        w477 = T3."Enabled" ("Disabled")
        n241 = property on="*Com Port" class="VISAName"("DisabledEnum"=w477) -> ()  [unwired: 2 in, 2 out]
        n242 = property on="*Baud Rate" class="CmbBox"("DisabledEnum"=w477) -> ()  [unwired: 2 in, 2 out]
        n243 = property on="*Timeout (sec)" class="DigNum (strict)"("DisabledEnum"=w477) -> ()  [unwired: 2 in, 2 out]
      }
      frame "Update Termination Character" {
        n244 = Unbundle By Name(w481) -> ("COM Port"=w480:refnum<visa-resource-name>)
        n245 = Variant To Data(Variant=w482, type=u8 10 ("termination char\n(0xA = '\\n' = LF)")) -> (data=w478:u8)  [unwired: 1 in, 1 out]
        n246 = property class="Instr"(reference=w480, "TermChar"=w478) -> ()  [unwired: 1 in, 2 out]
      }
      frame "Remote Open Port" {
        n247 = Variant To Data(Variant=w486, type="") -> (data=w484:string)  [unwired: 1 in, 1 out]
        n248 = case shown="\"\"" w484 {
          selector: w484 -> [_ w490]
          tunnel: w483 -> [_ w488]
          frame "" {
          }
          frame Default {
            n249 = local write "*Com Port"(w490) -> ()
            n250 = call "NextState.vi"("State"="Open Port", "Queue In"=w488) -> ()  [unwired: 8 in, 2 out]
          }
        }
      }
      frame "Open Port" {
        n251 = Unbundle By Name(w492) -> ("StartDelay"=w491:dbl)
        n252 = Match Pattern(string="*Com Port", regular expression="TCPIP") -> (offset past match=w493:i32)  [unwired: 1 in, 3 out]
        n253 = case shown="-1" w493 {
          tunnel: [w507 w512] -> w505
          tunnel: [_ w511] -> w501
          tunnel: "*Com Port" -> [w507 w513]
          tunnel: w491 -> [_ w508]
          frame Default {
            # "TCP Connection"
          }
          frame -1 {
            w524 = u16 0 items=["None", "XON/XOFF", "RTS/CTS", "XON/XOFF & RTS/CTS", "DTR/DSR", "XON/XOFF & DTR/DSR"] ("flow control (0:none)")
            n254 = Decimal String To Number(string="*Baud Rate", default (0L)=u32 0 ("default (0 I32)")) -> (number=w517:u32)  [unwired: 1 in, 1 out]
            n255 = call-poly "VISA Configure Serial Port"("VISA resource name"=w513, "timeout (10sec)"=u32 1000, "termination char\n(0xA = '\\n' = LF)"=u8 10 ("termination char\n(0xA = '\\n' = LF)"), "Enable Termination\nChar (T)"=TRUE ("Enable Termination\nChar (T)"), "baud rate (9600)"=w517, "flow control (0:none)"=w524) -> ("VISA resource name out"=w526:refnum<visa-resource-name>, "error out"=w510:errorcluster)  [unwired: 3 in, 5 out]
            n256 = call "Time Delay9"("error in (no error)"=w510, "Delay Time (s)"=w508) -> ("error out"=w509:errorcluster)  [unwired: 9 in]
            n257 = disable-structure shown="Enabled" {
              disable-tunnel: w526 -> [w531 w533]
              disable-tunnel: [w530 w533] -> w523
              disable-tunnel: [w529 w532] -> w522
              disable-tunnel: w509 -> [w528 w532]
              frame Disabled {
                n258 = VISA Open(error in (no error)=w528, VISA resource name=w531) -> (VISA resource name=w530:refnum<visa-resource-name>, error out=w529:errorcluster)  [unwired: 3 out]
              }
              frame Enabled {
              }
            }
            n259 = VISA Set I/O Buffer Size(VISA resource name=w523, size (4096)=u32 64000, error in (no error)=w522) -> (VISA resource name out=w520:refnum<visa-resource-name>, error out=w521:errorcluster)  [unwired: 1 out]
            n260 = property class="Instr"(reference=w520, error in=w521, "Timeout"=u32 1000 ("General Settings:Timeout Value")) -> (reference out=w512:refnum<visa-resource-name>, error out=w511:errorcluster)
          }
        }
        n261 = local write "Status"("Please Wait, Connecting to the AeroQuad..." ("Status")) -> ()
        n262 = call "NextState.vi"("State"="Lock User Controls", "Queue In"=w497) -> ("Queue Out"=w498:refnum<queue>)  [unwired: 8 in, 1 out]
        n263 = call "NextState.vi"("Error In"=w501, "State"="Check Connection", "Queue In"=w498) -> ()  [unwired: 7 in, 2 out]
        n264 = property on="Open Port" class="Bool"(error in=w501, "DisabledEnum"=T3."Disabled and Grayed Out" ("Disabled")) -> (error out=w496:errorcluster)  [unwired: 1 in, 1 out]
        n265 = Bundle By Name(cluster=w492, "COM Port"=w505, "Error"=w496) -> (w506:T2)
        n266 = local write "Sensors"(string[][] [] ("Sensors")) -> ()
      }
      frame "Check Connection" {
        n267 = Unbundle By Name(w541) -> ("COM Port"=w537:refnum<visa-resource-name>, "Version"=w545:string)
        n268 = call "NextState.vi"("State"="Connect", "Queue In"=w543) -> ()  [unwired: 8 in, 2 out]
        n269 = while {
          tunnel: w537 -> [w558]
          tunnel: w545 -> [w557]
          shift-right: [w555] -> w535
          shift-left: errorcluster {"status"=FALSE, "code"=0, "source"=""} ("error out") -> [w556]
          tunnel: "*Timeout (sec)" -> [w550]
          shift-right: [w547] -> _
          shift-left: TRUE -> [w548]
          tunnel: [w546] -> _
          i -> [w546]
          stop <- w547 stop-if-true
          n270 = VISA Write(VISA resource name=w558, write buffer=w557, error in (no error)=w556) -> (VISA resource name out=w551:refnum<visa-resource-name>, error out=w559:errorcluster)  [unwired: 1 out]
          n271 = call "Time Delay4"("error in (no error)"=w559) -> ("error out"=w552:errorcluster)  [unwired: 1 in, 9 out]
          n272 = VISA Read(VISA resource name=w551, byte count=u32 1024, error in (no error)=w552) -> (VISA resource name out=w553:refnum<visa-resource-name>, error out=w554:errorcluster)  [unwired: 2 out]
          n273 = case shown="Error" w554 {
            selector: w554 -> [w561 w564]
            tunnel: [w561 w562] -> w555
            tunnel: w553 -> [_ _]
            tunnel: w550 -> [_ w567]
            tunnel: [TRUE ("Time has Elapsed") w566] -> w547
            tunnel: w548 -> [_ w563]
            frame No Error {
            }
            frame Error {
              n274 = call "Elapsed Time"("Time Target (s)"=w567, "Reset"=w563) -> ("Time has Elapsed"=w566:bool, "error out"=w565:errorcluster)  [unwired: 10 in, 6 out]
              n275 = Select(t=w564, s=w566, f=w565) -> (s? t:f=w562:errorcluster)
            }
          }
        }
        n276 = call "Time Delay"("error in (no error)"=w535, "Delay Time (s)"=0.0) -> ("error out"=w534:errorcluster)  [unwired: 9 out]
        n277 = Bundle By Name(cluster=w541, "Error"=w534) -> (w540:T2)
      }
      frame "Connect" {
        n278 = Unbundle By Name(w597) -> ("COM Port"=w577:refnum<visa-resource-name>, "StopTelem"=w578:string, "Version"=w579:string)
        n279 = VISA Write(VISA resource name=w577, write buffer=w578) -> (VISA resource name out=w574:refnum<visa-resource-name>, error out=w573:errorcluster)  [unwired: 1 in, 1 out]
        n280 = call "Time Delay8"("error in (no error)"=w573) -> ("error out"=w572:errorcluster)  [unwired: 10 in]
        n281 = VISA Flush I/O Buffer(VISA resource name=w574, error in (no error)=w572) -> (VISA resource name out=w575:refnum<visa-resource-name>, error out=w576:errorcluster)  [unwired: 1 in]
        n282 = VISA Write(VISA resource name=w575, write buffer=w579, error in (no error)=w576) -> (VISA resource name out=w586:refnum<visa-resource-name>, error out=w585:errorcluster)  [unwired: 1 out]
        n283 = VISA Read(VISA resource name=w586, byte count=u32 1024, error in (no error)=w585) -> (VISA resource name out=w583:refnum<visa-resource-name>, read buffer=w580:string, error out=w584:errorcluster)  [unwired: 1 out]
        n284 = Decimal String To Number(string=w580) -> (number=w581:i32)  [unwired: 2 in, 1 out]
        n285 = for {
          N: w581 -> [_]
          tunnel: w583 -> [w608]
          shift-right: [w605] -> w593
          shift-left: w584 -> [w606]
          tunnel: [w601] -> w591 mode=indexing
          tunnel: [w600] -> w590 mode=indexing
          tunnel: [w599] -> w587 mode=indexing
          tunnel: [w598] -> w571
          n286 = VISA Read(VISA resource name=w608, byte count=u32 1024, error in (no error)=w606) -> (VISA resource name out=w598:refnum<visa-resource-name>, read buffer=w604:string, error out=w605:errorcluster)  [unwired: 1 out]
          n287 = Match Pattern(string=w604, regular expression=":") -> (before substring=w601:string, after substring=w602:string)  [unwired: 1 in, 2 out]
          n288 = call <vilib>:"Trim Whitespace.vi"("string"=w602) -> ("trimmed string"=w600:string)  [unwired: 1 in]
          n289 = Build Array(w601, w600) -> (w599:string[])
        }
        n290 = local read "*Timeout (sec)"() -> (w569:dbl)
        n291 = Multiply(x=w569, y=1000.0) -> (x*y=w570:dbl)
        n292 = property class="Instr"(reference=w571, "General Settings:Timeout Value"=w570) -> ()  [unwired: 1 in, 2 out]
        n293 = Unbundle By Name(w593) -> ("status"=w592:bool)
        n294 = property on="Sensors" class="Tbl (strict)"("Row Headers[]"=w591) -> ()  [unwired: 2 in, 2 out]
        n295 = Build Array(w590) -> (w589:string[][])
        n296 = Not(x=w592) -> (.not. x?=w594:bool)
        n297 = case shown="True" w594 {
          tunnel: w595 -> [_ w615]
          frame False {
          }
          frame True {
            n298 = call "NextStates.vi"("States"=string[] ["Update Parameters", "Unlock Controls", "Save Comm Controls", "Lock Comm Controls", "Unlock User Controls"], "Queue In"=w615) -> ("Queue Out"=w611:refnum<queue>)  [unwired: 8 in, 1 out]
            n299 = call "NextState.vi"("Data"="Connected to the AeroQuad!", "State"="Status", "Queue In"=w611) -> ("Queue Out"=w610:refnum<queue>)  [unwired: 7 in, 1 out]
            n300 = call <vilib>:"Beep.vi"() -> ()  [unwired: 12 in]
            n301 = call "NextState.vi"("State"="Load SubPanel", "Queue In"=w610) -> ()  [unwired: 8 in, 2 out]
          }
        }
        n302 = Transpose 2D Array(2D array=w589) -> (transposed array=→"Sensors":string[][])
        n303 = Bundle By Name(cluster=w597, "Config"=w587, "Connected"=w594, "Error"=w593) -> (w596:T2)
      }
      frame "Request Telemetry", "Send Command" {
        # "In a telemetry query, a command will be sent\nfirst, then a telemetry request."
        n304 = Unbundle By Name(w625) -> ("oldTelem"=w616:string, "Connected"=w622:bool, "COM Port"=w626:refnum<visa-resource-name>)
        n305 = case shown="True" w622 {
          tunnel: w626 -> [_ w632]
          tunnel: w623 -> [_ w635]
          tunnel: [_ w634] -> w621
          tunnel: w620 -> [w627 _]
          tunnel: w619 -> [w629 _]
          tunnel: [_ w633] -> w618
          tunnel: [_ w631] -> w617
          tunnel: w616 -> [_ w631]
          frame False {
            n306 = Flush Queue(queue=w627) -> (queue out=w628:refnum<queue>)  [unwired: 1 in, 2 out]
            n307 = case shown="\"Send Command\"" w629 {
              tunnel: w628 -> [_ _]
              frame Default {
              }
              frame "Send Command" {
                n308 = One Button Dialog(message="The AeroQuad is not connected to the Configurator!\nErroneous messages may appear.") -> ()  [unwired: 1 in, 1 out]
              }
            }
          }
          frame True {
            n309 = Variant To Data(Variant=w635, type="") -> (data=w633:string)  [unwired: 1 in, 1 out]
            n310 = VISA Write(VISA resource name=w632, write buffer=w633) -> (error out=w634:errorcluster)  [unwired: 1 in, 2 out]
          }
        }
        n311 = Bundle By Name(cluster=w625, "oldCmd"=w617, "oldTelem"=w618, "Error"=w621) -> (w624:T2)
      }
      frame "Clear Serial Comm" {
        n312 = Unbundle By Name(w641) -> ("Connected"=w639:bool, "COM Port"=w642:refnum<visa-resource-name>, "StopTelem"=w637:string)
        n313 = case shown="True" w639 {
          tunnel: w642 -> [_ w651]
          tunnel: [_ w648] -> w638
          tunnel: w637 -> [_ w647]
          frame False {
          }
          frame True {
            n314 = VISA Write(VISA resource name=w651, write buffer=w647) -> (VISA resource name out=w645:refnum<visa-resource-name>, error out=w649:errorcluster)  [unwired: 1 in, 1 out]
            n315 = call "Time Delay3"("error in (no error)"=w649, "Delay Time (s)"=0.25) -> ("error out"=w644:errorcluster)  [unwired: 9 in]
            n316 = VISA Flush I/O Buffer(VISA resource name=w645, error in (no error)=w644) -> (VISA resource name out=w646:refnum<visa-resource-name>, error out=w643:errorcluster)  [unwired: 1 in]
            n317 = disable-structure shown="Enabled" {
              disable-tunnel: [w659 _] -> w648
              disable-tunnel: w647 -> [w658 _]
              disable-tunnel: w646 -> [w653 _]
              disable-tunnel: w643 -> [w652 _]
              frame Enabled {
                n318 = VISA Write(VISA resource name=w653, write buffer=w658, error in (no error)=w652) -> (VISA resource name out=w654:refnum<visa-resource-name>, error out=w656:errorcluster)  [unwired: 1 out]
                n319 = call "Time Delay5"("error in (no error)"=w656, "Delay Time (s)"=0.25) -> ("error out"=w655:errorcluster)  [unwired: 9 in]
                n320 = VISA Flush I/O Buffer(VISA resource name=w654, error in (no error)=w655) -> (error out=w659:errorcluster)  [unwired: 1 in, 1 out]
              }
              frame Disabled {
              }
            }
          }
        }
        n321 = Bundle By Name(cluster=w641, "Error"=w638) -> (w640:T2)
      }
      frame "Reconnect" {
        n322 = in-place {
          in-place-border: [w670] -> w662
          n323 = in-place-cluster #3(w665) -> ("Error"=w672:errorcluster)
          n324 = call "ReconnectDialog.vi"("error in"=w672) -> ("error out"=w671:errorcluster, "AbortConnection"=w670:bool)  [unwired: 9 in]
          n325 = in-place-cluster #3("Error"=w671) -> (w664:T2)
        }
        n326 = case shown="True" w662 {
          tunnel: w663 -> [w667 w669]
          tunnel: [w667 w669] -> w661
          tunnel: ["Unlock User Controls" "Open Port"] -> w660
          frame False {
          }
          frame True {
          }
        }
        n327 = call "NextState.vi"("State"=w660, "Queue In"=w661) -> ()  [unwired: 8 in, 2 out]
      }
      frame "Disconnect" {
        n328 = Unbundle By Name(w685) -> ("COM Port"=w675:refnum<visa-resource-name>, "StopTelem"=w673:string)
        n329 = call "NextState.vi"("State"="Lock Controls", "Queue In"=w681) -> ("Queue Out"=w679:refnum<queue>)  [unwired: 8 in, 1 out]
        n330 = VISA Write(VISA resource name=w675, write buffer=w673) -> (VISA resource name out=w674:refnum<visa-resource-name>)  [unwired: 1 in, 2 out]
        n331 = VISA Close(VISA resource name=w674) -> ()  [unwired: 1 in, 1 out]
        n332 = call "PriorityState.vi"("Data"="Disconnected from AeroQuad", "State"="Status", "Queue In"=w679) -> ("Queue Out"=w678:refnum<queue>)  [unwired: 7 in, 1 out]
        n333 = call "NextState.vi"("State"="Unlock Comm Controls", "Queue In"=w678) -> ()  [unwired: 8 in, 2 out]
        n334 = Bundle By Name(cluster=w685, "Connected"=FALSE) -> (w684:T2)
      }
      frame "Update Timeout" {
        n335 = Unbundle By Name(w686) -> ("COM Port"=w690:refnum<visa-resource-name>)
        n336 = Variant To Data(Variant=w689, type=u32 0 ("General Settings:Timeout Value")) -> (data=w687:u32)  [unwired: 1 in, 1 out]
        n337 = property class="Instr"(reference=w690, "Timeout"=w687) -> ()  [unwired: 1 in, 2 out]
      }
      frame "Default Timeout" {
        n338 = Unbundle By Name(w695) -> ("COM Port"=w696:refnum<visa-resource-name>)
        n339 = local read "*Timeout (sec)"() -> (w692:dbl)
        n340 = Compound Arithmetic op=MULTIPLY(w692, 1000.0 ("value")) -> (w694:dbl)
        n341 = To Unsigned Long Integer(number=w694) -> (unsigned 32bit integer=w691:u32)
        n342 = property class="Instr"(reference=w696, "Timeout"=w691) -> ()  [unwired: 1 in, 2 out]
      }
      frame "--- Parameters ---" {
      }
      frame "Parameter Check" {
        # "Validate data in text table."
        n343 = local read "Parameter Type"() -> (w704:i32)
        n344 = Unbundle By Name(w711) -> ("Parameters"=w707:string[][][])
        n345 = Index Array(array=w707, index (dim 0)=w704, index (dim 2)=1 ("disabled index (col)")) -> (element=w709:string[])  [unwired: 1 in]
        n346 = Index Array(array="Parameter Check", index (col)=0 ("disabled index (col)")) -> (element=w702:string[])  [unwired: 1 in]
        n347 = Split 1D Array(array=w709, index=2) -> (second subarray=w706:string[])  [unwired: 1 out]
        n348 = for {
          tunnel: w706 -> [w713] mode=indexing
          tunnel: [w712] -> w700 mode=indexing
          tunnel: w702 -> [w718] mode=indexing
          n349 = call <vilib>:"Trim Whitespace.vi"("string"=w718) -> ("trimmed string"=w717:string)  [unwired: 1 in]
          n350 = Search and Replace String(replace all?=TRUE ("replace all? (F)"), input string=w717, search string=",", replace string="." ("replace string (\"\")")) -> (result string=w722:string)  [unwired: 4 in, 3 out]
          n351 = Fract/Exp String To Number(use system decimal point (T)=FALSE, string=w722) -> (offset past number=w716:i32, number=w724:dbl)  [unwired: 2 in]
          n352 = Greater Than 0?(x=w716) -> (x > 0?=w715:bool)
          n353 = Format Value(format string="%#g", value (0)=w724) -> (output string=w714:string)  [unwired: 1 in]
          n354 = Select(t=w714, s=w715, f=w713) -> (s? t:f=w712:string)
        }
        n355 = Replace Array Subset(array="Parameter Check", new element=w700, index (col)=0 ("disabled index (col)")) -> (w703:string[][])  [unwired: 1 in]
        n356 = local write "Parameter Check"(w703) -> ()
        n357 = property on="Parameter Check" class="Tbl (strict)"("Selection Start"=T5 {"Row"=10, "Column"=10} ("Selection Size")) -> ()  [unwired: 2 in, 2 out]
      }
      frame "Parameter Type" {
        # "Load paramater values into table"
        # "Load paramater names into table"
        n358 = Unbundle By Name(w743) -> ("Parameters"=w742:string[][][])
        n359 = Index Array(array=w742, index (dim 0)="Parameter Type", index (dim 2)=1 ("disabled index (col)")) -> (element=w737:string[])  [unwired: 1 in]
        n360 = Split 1D Array(array=w737, index=2) -> (second subarray=w731:string[])  [unwired: 1 out]
        n361 = Index Array(array=w742, index (dim 0)="Parameter Type", index (dim 2)=0 ("disabled index (col)")) -> (element=w735:string[])  [unwired: 1 in]
        n362 = Split 1D Array(array=w735, index=2) -> (second subarray=w727:string[])  [unwired: 1 out]
        n363 = Search 1D Array(1D array=w727, element="") -> (index of element=w729:i32)  [unwired: 1 in]
        n364 = case shown="..0" w729 {
          selector: w729 -> [_ w746]
          tunnel: [w745 w746] -> w728
          tunnel: w727 -> [w744 _]
          frame ..0 {
            n365 = Array Size(array=w744) -> (size(s)=w745:i32)
          }
          frame Default {
          }
        }
        n366 = property on="Parameter Check" class="Tbl (strict)"("Selection Start"=T6 {"Row"=10, "Column"=10} ("Index Values"), "Row Headers[]"=w727) -> ()  [unwired: 2 in, 2 out]
        n367 = Split 1D Array(array=w731, index=w728) -> (first subarray=w732:string[])  [unwired: 1 out]
        n368 = Build Array(w732) -> (w739:string[][])
        n369 = Transpose 2D Array(2D array=w739) -> (transposed array=w738:string[][])
        n370 = local write "Parameter Check"(w738) -> ()
      }
      frame "Update Parameters" {
        n371 = Unbundle By Name(w759) -> ("Parameters"=w757:string[][][], "COM Port"=w756:refnum<visa-resource-name>, "Error"=w747:errorcluster)
        n372 = call "Time Delay7"("error in (no error)"=w747) -> ("error out"=w748:errorcluster)  [unwired: 10 in]
        n373 = for {
          tunnel: w757 -> [w768] mode=indexing
          tunnel: w756 -> [w776]
          shift-right: [w772] -> w755
          shift-left: w748 -> [w773]
          tunnel: [w767] -> w754 mode=indexing
          tunnel: [w762] -> w753 mode=indexing
          n374 = Index Array(array=w768, index (col)=0 ("disabled index (col)")) -> (element=w780:string[])  [unwired: 1 in]
          n375 = Search 1D Array(1D array=w780, element="Telemetry") -> (index of element=w778:i32)  [unwired: 1 in]
          n376 = Index Array(array=w768, index (row)=w778, index (col)=1 ("disabled index (col)")) -> (element=w775:string)
          n377 = VISA Write(VISA resource name=w776, write buffer=w775, error in (no error)=w773) -> (VISA resource name out=w764:refnum<visa-resource-name>, error out=w766:errorcluster)  [unwired: 1 out]
          n378 = call "Time Delay2"("error in (no error)"=w766) -> ("error out"=w765:errorcluster)  [unwired: 10 in]
          n379 = VISA Read(VISA resource name=w764, byte count=u32 1024, error in (no error)=w765) -> (read buffer=w760:string, error out=w772:errorcluster)  [unwired: 2 out]
          n380 = call "RemoveTrailingComma.vi"("Input String"=w760) -> ("Output String"=w761:string)  [unwired: 8 in]
          n381 = Spreadsheet String To Array(delimiter (Tab)=",", format string="%s", spreadsheet string=w761, array type (2D Dbl)=string[] []) -> (array=w763:string[])
          n382 = for {
            shift-right: [w791] -> w767
            shift-left: w768 -> [w792]
            tunnel: w763 -> [w783] mode=indexing
            tunnel: [w782] -> w762 mode=indexing
            i -> [w788]
            n383 = Fract/Exp String To Number(use system decimal point (T)=FALSE, string=w783) -> (number=w785:dbl)  [unwired: 2 in, 1 out]
            n384 = Format Value(format string="%#g", value (0)=w785) -> (output string=w782:string)  [unwired: 1 in]
            n385 = Compound Arithmetic op=ADD(2 ("disabled index (row)"), w788) -> (w787:i32)
            n386 = Replace Array Subset(array=w792, new element=w782, index (row)=w787, index (col)=1 ("disabled index (col)")) -> (w791:string[][])
          }
        }
        n387 = local read "Parameter Type"() -> (w752:i32)
        n388 = Index Array(array=w753, index (row)=w752) -> (element=w751:string[])  [unwired: 1 in]
        n389 = Build Array(w751) -> (w750:string[][])
        n390 = Transpose 2D Array(2D array=w750) -> (transposed array=w749:string[][])
        n391 = local write "Parameter Check"(w749) -> ()
        n392 = Bundle By Name(cluster=w759, "Parameters"=w754, "Error"=w755) -> (w758:T2)
      }
      frame "Update Parameter" {
        n393 = local read "Parameter Type"() -> (w800:i32)
        n394 = Unbundle By Name(w821) -> ("Parameters"=w801:string[][][], "COM Port"=w819:refnum<visa-resource-name>, "Error"=w818:errorcluster)
        n395 = Index Array(array=w801, index (dim 0)=w800) -> (element=w802:string[][])  [unwired: 2 in]
        n396 = Index Array(array=w802, index (col)=0 ("disabled index (col)")) -> (element=w815:string[])  [unwired: 1 in]
        n397 = Search 1D Array(1D array=w815, element="Telemetry") -> (index of element=w813:i32)  [unwired: 1 in]
        n398 = Index Array(array=w802, index (row)=w813, index (col)=1 ("disabled index (col)")) -> (element=w811:string)
        n399 = VISA Write(VISA resource name=w819, write buffer=w811, error in (no error)=w818) -> (VISA resource name out=w804:refnum<visa-resource-name>, error out=w806:errorcluster)  [unwired: 1 out]
        n400 = call "Time Delay6"("error in (no error)"=w806) -> ("error out"=w805:errorcluster)  [unwired: 10 in]
        n401 = VISA Read(VISA resource name=w804, byte count=u32 1024, error in (no error)=w805) -> (read buffer=w794:string, error out=w817:errorcluster)  [unwired: 2 out]
        n402 = call "RemoveTrailingComma.vi"("Input String"=w794) -> ("Output String"=w793:string)  [unwired: 8 in]
        n403 = Spreadsheet String To Array(delimiter (Tab)=",", format string="%s", spreadsheet string=w793, array type (2D Dbl)=string[] []) -> (array=w803:string[])
        n404 = for {
          shift-right: [w831] -> w798
          shift-left: w802 -> [w832]
          tunnel: w803 -> [w823] mode=indexing
          tunnel: [w822] -> w797 mode=indexing
          i -> [w828]
          n405 = Fract/Exp String To Number(use system decimal point (T)=FALSE, string=w823) -> (number=w825:dbl)  [unwired: 2 in, 1 out]
          n406 = Format Value(format string="%#g", value (0)=w825) -> (output string=w822:string)  [unwired: 1 in]
          n407 = Compound Arithmetic op=ADD(2 ("disabled index (row)"), w828) -> (w827:i32)
          n408 = Replace Array Subset(array=w832, new element=w822, index (row)=w827, index (col)=1 ("disabled index (col)")) -> (w831:string[][])
        }
        n409 = Build Array(w797) -> (w796:string[][])
        n410 = Transpose 2D Array(2D array=w796) -> (transposed array=w795:string[][])
        n411 = local write "Parameter Check"(w795) -> ()
        n412 = Replace Array Subset(array=w801, new element=w798, index (dim 0)=w800) -> (w799:string[][][])  [unwired: 2 in]
        n413 = Bundle By Name(cluster=w821, "Parameters"=w799, "Error"=w817) -> (w820:T2)
      }
      frame "Upload" {
        w833 = T3."Disabled and Grayed Out" ("Disabled")
        n414 = Flush Queue(queue=w835) -> (queue out=w834:refnum<queue>)  [unwired: 1 in, 2 out]
        n415 = Unbundle By Name(w881) -> ("Parameters"=w856:string[][][])
        n416 = local read "Parameter Check"() -> (w878:string[][])
        n417 = local read "Parameter Type"() -> (w855:i32)
        n418 = call "NextState.vi"("Data"="Uploading to AeroQuad", "State"="Status", "Queue In"=w834) -> ("Queue Out"=w845:refnum<queue>)  [unwired: 7 in, 1 out]
        n419 = Index Array(array=w878, index (col)=0 ("disabled index (col)")) -> (element=w861:string[])  [unwired: 1 in]
        n420 = call "NextState.vi"("State"="Clear Serial Comm", "Queue In"=w845) -> ("Queue Out"=w838:refnum<queue>)  [unwired: 8 in, 1 out]
        n421 = Index Array(array=w856, index (dim 0)=w855, index (dim 2)=0 ("disabled index (row)")) -> (element=w869:string[])  [unwired: 1 in]
        n422 = Array To Spreadsheet String(delimiter (Tab)=";", array=w861, 3:"%s" ("format string")) -> (spreadsheet string=w850:string)
        n423 = Search 1D Array(1D array=w869, element="Command") -> (index of element=w858:i32)  [unwired: 1 in]
        n424 = Match Pattern(string=w850, regular expression=";;") -> (before substring=w852:string)  [unwired: 4 out]
        n425 = Index Array(array=w856, index (dim 0)=w855, index (dim 1)=w858, index (dim 2)=1 ("disabled index (col)")) -> (element=w872:string)
        n426 = call "NextState.vi"("State"="Default Timeout", "Queue In"=w838) -> ("Queue Out"=w837:refnum<queue>)  [unwired: 8 in, 1 out]
        n427 = Match Pattern(string=w852, regular expression="\r\n") -> (before substring=w862:string)  [unwired: 4 out]
        n428 = Format Into String(format string="%s%s;", w872, w862) -> (resulting string=w871:string)  [unwired: 2 in, 1 out]
        n429 = Array To Spreadsheet String(delimiter (Tab)=",", array=w861, 3:"%s" ("format string")) -> (spreadsheet string=w847:string)
        n430 = Search 1D Array(1D array=w869, element="Telemetry") -> (index of element=w854:i32)  [unwired: 1 in]
        n431 = call "NextState.vi"("Data"=w871, "State"="Send Command", "Queue In"=w837) -> ("Queue Out"=w867:refnum<queue>)  [unwired: 7 in, 1 out]
        n432 = Index Array(array=w856, index (dim 0)=w855, index (dim 1)=w854, index (dim 2)=1 ("disabled index (col)")) -> (element=w849:string)
        n433 = Match Pattern(string=w847, regular expression=",,") -> (before substring=w848:string)  [unwired: 4 out]
        n434 = Match Pattern(string=w848, regular expression="\r\n") -> (before substring=w844:string)  [unwired: 4 out]
        n435 = call "NextState.vi"("Data"=w849, "State"="Request Telemetry", "Queue In"=w867) -> ("Queue Out"=w866:refnum<queue>)  [unwired: 7 in, 1 out]
        n436 = call "NextState.vi"("Data"=w844, "State"="Verify Upload", "Queue In"=w866) -> ("Queue Out"=w841:refnum<queue>)  [unwired: 7 in, 1 out]
        n437 = call "NextState.vi"("State"="Update Parameter", "Queue In"=w841) -> ("Queue Out"=w840:refnum<queue>)  [unwired: 8 in, 1 out]
        n438 = property on="Upload" class="Bool"("DisabledEnum"=w833) -> ()  [unwired: 2 in, 2 out]
        n439 = property on="Parameter Type" class="Ring (strict)"("DisabledEnum"=w833) -> ()  [unwired: 2 in, 2 out]
        n440 = call "NextState.vi"("State"="Load SubPanel", "Queue In"=w840) -> ()  [unwired: 8 in, 2 out]
      }
      frame "Update Tool Tip" {
        n441 = Unbundle By Name(w890) -> ("ParamDesc"=w889:string[][])
        n442 = Variant To Data(Variant=w892, type=0) -> (data=w887:i32)  [unwired: 1 in, 1 out]
        n443 = local read "Parameter Type"() -> (w888:i32)
        n444 = Add(x=w887, y=2) -> (x+y=w885:i32)
        n445 = Index Array(array=w889, index (row)=w888, index (col)=w885) -> (element=w886:string)
        n446 = property on="Parameter Check" class="Tbl (strict)"("TipStrip"=w886) -> ()  [unwired: 2 in, 2 out]
      }
      frame "Next Parameter" {
        n447 = property on="Parameter Check" class="Tbl (strict)"() -> ("EditPos"=w904:T5, "Value"=w901:string[][])  [unwired: 2 in, 2 out]
        n448 = Array Size(array=w901) -> (size(s)=w900:i32[])
        n449 = call "NextState.vi"("State"="Update Tool Tip", "Queue In"=w894) -> ()  [unwired: 8 in, 2 out]
        n450 = Index Array(array=w900) -> (element=w899:i32)  [unwired: 1 in]
        n451 = Unbundle By Name(w904) -> ("Row"=w903:i32)
        n452 = Increment(x=w903) -> (x+1=w897:i32)
        n453 = Equal?(x=w897, y=w899) -> (x = y?=w898:bool)
        n454 = Select(t=0, s=w898, f=w897) -> (s? t:f=w895:i32)
        n455 = Bundle By Name(cluster=w904, "Row"=w895) -> (w902:T5)
        n456 = property on="Parameter Check" class="Tbl (strict)"("EditPos"=w902) -> ()  [unwired: 2 in, 2 out]
      }
      frame "--- Telemetry ---" {
      }
      frame "Read Continuous" {
        # "To send data continously to a subPanel, have queue message sent to main GUI to this state"
        n457 = Unbundle By Name(w911) -> ("SubPanelQueue"=w909:refnum<queue>, "COM Port"=w912:refnum<visa-resource-name>, "Connected"=w907:bool)
        n458 = case shown="True" w907 {
          tunnel: w912 -> [_ w926]
          tunnel: w911 -> [w913 w925]
          tunnel: [w913 w922] -> w910
          tunnel: w909 -> [_ w918]
          tunnel: w908 -> [_ w916]
          frame False {
          }
          frame True {
            n459 = VISA Read(VISA resource name=w926, byte count=u32 1024) -> (read buffer=w915:string, error out=w924:errorcluster)  [unwired: 1 in, 2 out]
            n460 = Bundle By Name(cluster=w925, "Error"=w924) -> (w922:T2)
            n461 = call "NextState.vi"("State"="Read Continuous", "Queue In"=w916) -> ()  [unwired: 8 in, 2 out]
            n462 = call "RemoveTrailingComma.vi"("Input String"=w915) -> ("Output String"=w914:string)  [unwired: 8 in]
            n463 = Spreadsheet String To Array(delimiter (Tab)=",", format string="%s", spreadsheet string=w914) -> (array=w919:dbl[][])  [unwired: 1 in]
            n464 = call "NextState.vi"("Data"=w919, "State"="Update", "Queue In"=w918) -> ()  [unwired: 7 in, 2 out]
          }
        }
      }
      frame "Read Continuous Binary" {
        # "To send data continously to a subPanel, have queue message sent to main GUI to this state"
        n465 = Unbundle By Name(w932) -> ("SubPanelQueue"=w930:refnum<queue>, "COM Port"=w933:refnum<visa-resource-name>, "Connected"=w928:bool)
        n466 = case shown="True" w928 {
          tunnel: w933 -> [_ w944]
          tunnel: w932 -> [w934 w943]
          tunnel: [w934 w940] -> w931
          tunnel: w930 -> [_ w939]
          tunnel: w929 -> [_ w937]
          frame False {
          }
          frame True {
            n467 = VISA Read(VISA resource name=w944, byte count=u32 1024) -> (read buffer=w936:string, error out=w942:errorcluster)  [unwired: 1 in, 2 out]
            n468 = String To Byte Array(string=w936) -> (unsigned byte array=w935:u8[])
            n469 = Bundle By Name(cluster=w943, "Error"=w942) -> (w940:T2)
            n470 = call "NextState.vi"("State"="Read Continuous Binary", "Queue In"=w937) -> ()  [unwired: 8 in, 2 out]
            n471 = call "NextState.vi"("Data"=w935, "State"="Update", "Queue In"=w939) -> ()  [unwired: 7 in, 2 out]
          }
        }
      }
      frame "Read Once" {
        n472 = Unbundle By Name(w949) -> ("SubPanelQueue"=w947:refnum<queue>, "COM Port"=w950:refnum<visa-resource-name>, "Connected"=w946:bool)
        n473 = case shown="True" w946 {
          tunnel: w950 -> [_ w962]
          tunnel: w949 -> [w951 w961]
          tunnel: [w951 w958] -> w948
          tunnel: w947 -> [_ w954]
          frame False {
          }
          frame True {
            n474 = VISA Read(VISA resource name=w962, byte count=u32 1024) -> (read buffer=w952:string, error out=w960:errorcluster)  [unwired: 1 in, 2 out]
            n475 = Bundle By Name(cluster=w961, "Error"=w960) -> (w958:T2)
            n476 = call "RemoveTrailingComma.vi"("Input String"=w952) -> ("Output String"=w953:string)  [unwired: 8 in]
            n477 = Spreadsheet String To Array(delimiter (Tab)=",", format string="%s", spreadsheet string=w953) -> (array=w955:dbl[][])  [unwired: 1 in]
            n478 = call "NextState.vi"("Data"=w955, "State"="Update", "Queue In"=w954) -> ()  [unwired: 7 in, 2 out]
          }
        }
      }
      frame "Read Serial Monitor Data" {
        n479 = Unbundle By Name(w968) -> ("SubPanelQueue"=w966:refnum<queue>, "COM Port"=w969:refnum<visa-resource-name>, "Connected"=w965:bool)
        n480 = case shown="True" w965 {
          tunnel: w969 -> [_ w979]
          tunnel: w968 -> [w970 w974]
          tunnel: [w970 w973] -> w967
          tunnel: w966 -> [_ w977]
          tunnel: w964 -> [_ w971]
          frame False {
          }
          frame True {
            n481 = VISA Read(VISA resource name=w979, byte count=u32 1024) -> (read buffer=w978:string, error out=w975:errorcluster)  [unwired: 1 in, 2 out]
            n482 = Unbundle By Name(w975) -> ("code"=w976:i32)
            n483 = case shown="0" w976 {
              tunnel: w978 -> [_ _ w986]
              tunnel: w977 -> [_ _ w988]
              tunnel: [w981 w982 w987] -> w972
              tunnel: w975 -> [w981 w983 _]
              tunnel: w971 -> [_ _ w985]
              frame Default {
              }
              frame -1073807339, -1073807252, 56 {
                n484 = call <vilib>:"Clear Errors.vi"("error in (no error)"=w983) -> ("error out"=w982:errorcluster)  [unwired: 6 out]
              }
              frame 0 {
                n485 = call "NextState.vi"("State"="Read Serial Monitor Data", "Queue In"=w985) -> ()  [unwired: 8 in, 2 out]
                n486 = call "NextState.vi"("Data"=w986, "State"="Update", "Queue In"=w988) -> ("Error Out"=w987:errorcluster)  [unwired: 7 in, 1 out]
              }
            }
            n487 = Bundle By Name(cluster=w974, "Error"=w972) -> (w973:T2)
          }
        }
      }
      frame "Verify Upload" {
        n488 = Variant To Data(Variant=w993, type="") -> (data=w991:string)  [unwired: 1 in, 1 out]
        n489 = Unbundle By Name(w996) -> ("COM Port"=w997:refnum<visa-resource-name>, "Connected"=w994:bool)
        n490 = case shown="True" w994 {
          tunnel: w997 -> [_ w1012]
          tunnel: w996 -> [w998 w1011]
          tunnel: [w998 w1010] -> w995
          tunnel: w991 -> [_ w1003]
          tunnel: w990 -> [_ w1008]
          frame False {
          }
          frame True {
            n491 = call "RemoveTrailingComma.vi"("Input String"=w1003) -> ("Output String"=w999:string)  [unwired: 8 in]
            n492 = VISA Read(VISA resource name=w1012, byte count=u32 1024) -> (VISA resource name out=w1007:refnum<visa-resource-name>, read buffer=w1004:string, error out=w1005:errorcluster)  [unwired: 1 in, 1 out]
            n493 = call "RemoveTrailingComma.vi"("Input String"=w1004) -> ("Output String"=w1001:string)  [unwired: 8 in]
            n494 = call "ConvertNumericString.vi"("Input"=w999) -> ("Output"=w1002:string)  [unwired: 8 in]
            n495 = call "ConvertNumericString.vi"("Input"=w1001) -> ("Output"=w1000:string)  [unwired: 8 in]
            n496 = Equal?(x=w1002, y=w1000) -> (x = y?=w1009:bool)
            n497 = case shown="False" w1009 {
              tunnel: w1001 -> [w1019 _]
              tunnel: w999 -> [w1020 _]
              tunnel: w1008 -> [w1014 w1026]
              tunnel: w1007 -> [_ w1030]
              tunnel: [w1017 w1029] -> w1006
              tunnel: w1005 -> [w1017 w1028]
              frame False {
                n498 = Format Into String(format string="Parameter update was not successful.\nExpected Response:\n%s\n\nTry Again?\nReceived Response:\n%s", w1020, w1019) -> (resulting string=w1018:string)  [unwired: 2 in, 1 out]
                n499 = Two Button Dialog(message=w1018, 2:"Retry" ("T button name (\"OK\")")) -> (T button?=w1015:bool)  [unwired: 1 in]
                n500 = case shown="True" w1015 {
                  tunnel: w1014 -> [_ w1023]
                  frame False {
                  }
                  frame True {
                    n501 = call "PriorityState.vi"("State"="Retry Upload", "Queue In"=w1023) -> ()  [unwired: 8 in, 2 out]
                  }
                }
              }
              frame True {
                n502 = call "PriorityState.vi"("Data"="Upload successful!", "State"="Status", "Queue In"=w1026) -> ()  [unwired: 7 in, 2 out]
                n503 = VISA Write(VISA resource name=w1030, write buffer="W", error in (no error)=w1028) -> (error out=w1029:errorcluster)  [unwired: 2 out]
              }
            }
            n504 = Bundle By Name(cluster=w1011, "Error"=w1006, "previousValid"=w1003) -> (w1010:T2)
          }
        }
      }
      frame "Retry Upload" {
        n505 = Unbundle By Name(w1044) -> ("oldCmd"=w1042:string, "oldTelem"=w1031:string, "previousValid"=w1032:string)
        n506 = disable-structure shown="Disabled" {
          disable-tunnel: w1038 -> [w1046 w1047]
          disable-tunnel: [w1045 w1047] -> w1037
          frame Disabled {
            n507 = Flush Queue(queue=w1046) -> (queue out=w1045:refnum<queue>)  [unwired: 1 in, 2 out]
          }
          frame Enabled {
          }
        }
        n508 = call "NextState.vi"("Data"=w1042, "State"="Send Command", "Queue In"=w1037) -> ("Queue Out"=w1040:refnum<queue>)  [unwired: 7 in, 1 out]
        n509 = call "NextState.vi"("State"="Delay SubPanel", "Queue In"=w1040) -> ("Queue Out"=w1035:refnum<queue>)  [unwired: 8 in, 1 out]
        n510 = call "NextState.vi"("Data"=w1031, "State"="Request Telemetry", "Queue In"=w1035) -> ("Queue Out"=w1034:refnum<queue>)  [unwired: 7 in, 1 out]
        n511 = call "NextState.vi"("Data"=w1032, "State"="Verify Upload", "Queue In"=w1034) -> ("Queue Out"=w1036:refnum<queue>)  [unwired: 7 in, 1 out]
        n512 = disable-structure shown="Disabled" {
          disable-tunnel: w1036 -> [w1049 _]
          frame Disabled {
            n513 = call "NextState.vi"("State"="Update Parameter", "Queue In"=w1049) -> ()  [unwired: 8 in, 2 out]
          }
          frame Enabled {
          }
        }
      }
      frame "--- File Operations ---" {
      }
      frame "File Open" {
        n514 = call "File Dialog"("prompt"="Select AeroQuad Config File", "pattern (all files)"="*.aq", "pattern label"="AeroQuad Config") -> ("selected path"=w1055:path, "cancelled"=w1051:bool)  [unwired: 9 in, 2 out]
        n515 = case shown="False" w1051 {
          tunnel: w1055 -> [w1083 _]
          tunnel: w1053 -> [w1082 _]
          tunnel: w1054 -> [w1065 _]
          tunnel: w1053 -> [w1069 w1112]
          tunnel: [w1068 w1112] -> w1052
          frame False {
            w1059 = 0
            n516 = Unbundle By Name(w1082) -> ("ParameterName"=w1076:string[], "Parameters"=w1075:string[][][])
            n517 = Flush Queue(queue=w1065) -> (queue out=w1061:refnum<queue>)  [unwired: 1 in, 2 out]
            n518 = call <vilib>:"Open Config Data.vi"("configuration file path"=w1083) -> ("error out"=w1080:errorcluster, "refnum"=w1081:T1)  [unwired: 8 in, 1 out]
            n519 = call <vilib>:"Get Section Names.vi"("error in (no error)"=w1080, "refnum"=w1081) -> ("error out"=w1078:errorcluster, "section names"=w1077:string[], "refnum out"=w1079:T1)  [unwired: 7 in]
            n520 = for {
              tunnel: w1079 -> [w1097]
              shift-right: [w1085] -> w1072
              shift-left: w1078 -> [w1096]
              tunnel: w1077 -> [w1091] mode=indexing
              tunnel: w1076 -> [w1098]
              shift-right: [w1087] -> w1074
              shift-left: w1075 -> [w1089]
              tunnel: [w1084] -> w1071
              n521 = call <vilib>:"Get Key Names.vi"("section"=w1091, "error in (no error)"=w1096, "refnum"=w1097) -> ("error out"=w1086:errorcluster, "key names"=w1092:string[], "refnum out"=w1093:T1)  [unwired: 5 in, 1 out]
              n522 = Search 1D Array(1D array=w1098, element=w1091) -> (index of element=w1088:i32)  [unwired: 1 in]
              n523 = Index Array(array=w1089, index (dim 0)=w1088) -> (element=w1094:string[][])  [unwired: 2 in]
              n524 = Index Array(array=w1094, index (col)=0 ("disabled index (col)")) -> (element=w1090:string[])  [unwired: 1 in]
              n525 = for {
                tunnel: w1093 -> [w1111]
                tunnel: w1092 -> [w1108] mode=indexing
                tunnel: w1091 -> [w1110]
                tunnel: w1090 -> [w1109]
                shift-right: [w1102] -> w1087
                shift-left: w1089 -> [w1107]
                tunnel: w1088 -> [w1106]
                shift-right: [w1100] -> w1085
                shift-left: w1086 -> [w1101]
                tunnel: [w1099] -> w1084
                n526 = call-poly <vilib>:"Read Key.vi"("section"=w1110, "error in (no error)"=w1101, "key"=w1108, "refnum"=w1111) -> ("error out"=w1100:errorcluster, "value"=w1103:string, "refnum out"=w1099:T1)  [unwired: 4 in, 1 out]
                n527 = Search 1D Array(1D array=w1109, element=w1108) -> (index of element=w1104:i32)  [unwired: 1 in]
                n528 = Replace Array Subset(array=w1107, new element=w1103, index (dim 0)=w1106, index (dim 1)=w1104, index (dim 2)=1 ("disabled index (col)")) -> (w1102:string[][][])
              }
            }
            n529 = call "NextState.vi"("State"="Clear Serial Comm", "Queue In"=w1061) -> ("Queue Out"=w1064:refnum<queue>)  [unwired: 8 in, 1 out]
            n530 = call "NextState.vi"("State"="Default Timeout", "Queue In"=w1064) -> ("Queue Out"=w1062:refnum<queue>)  [unwired: 8 in, 1 out]
            n531 = call "NextState.vi"("State"="Parameter Type", "Queue In"=w1062) -> ("Queue Out"=w1066:refnum<queue>)  [unwired: 8 in, 1 out]
            n532 = call <vilib>:"Close Config Data.vi"("error in (no error)"=w1072, "refnum"=w1071) -> ("error out"=w1070:errorcluster)  [unwired: 8 in, 1 out]
            n533 = Bundle By Name(cluster=w1069, "Error"=w1070, "Parameters"=w1074) -> (w1068:T2)
            n534 = property on="Parameter Type" class="Ring (strict)"("Value"=w1059) -> ()  [unwired: 2 in, 2 out]
            n535 = call "NextState.vi"("Data"=w1059, "State"="File Upload", "Queue In"=w1066) -> ()  [unwired: 7 in, 2 out]
          }
          frame True {
          }
        }
      }
      frame "File Next" {
        n536 = Variant To Data(Variant=w1117, type=0) -> (data=w1114:i32)  [unwired: 1 in, 1 out]
        n537 = property on="Parameter Type" class="Ring (strict)"() -> ("NumItems"=w1119:u32)  [unwired: 2 in, 2 out]
        n538 = Increment(x=w1114) -> (x+1=w1113:i32)
        n539 = Less?(x=w1113, y=w1119) -> (x < y?=w1118:bool)
        n540 = case shown="True" w1118 {
          tunnel: w1113 -> [_ w1126]
          tunnel: w1115 -> [w1125 w1129]
          frame False {
            n541 = call "NextState.vi"("Data"="Finished loading AeroQuad configuration file." ("State"), "State"="Status", "Queue In"=w1125) -> ("Queue Out"=w1121:refnum<queue>)  [unwired: 7 in, 1 out]
            n542 = call "NextState.vi"("State"="Load SubPanel", "Queue In"=w1121) -> ()  [unwired: 8 in, 2 out]
          }
          frame True {
            n543 = local write "Parameter Type"(w1126) -> ()
            n544 = call "NextState.vi"("State"="Parameter Type", "Queue In"=w1129) -> ("Queue Out"=w1127:refnum<queue>)  [unwired: 8 in, 1 out]
            n545 = call "NextState.vi"("Data"=w1126, "State"="File Upload", "Queue In"=w1127) -> ()  [unwired: 7 in, 2 out]
          }
        }
      }
      frame "File Upload" {
        n546 = Variant To Data(Variant=w1132, type=0) -> (data=w1131:i32)  [unwired: 1 in, 1 out]
        n547 = Unbundle By Name(w1180) -> ("Parameters"=w1155:string[][][])
        n548 = local read "Parameter Check"() -> (w1177:string[][])
        n549 = Index Array(array=w1177, index (col)=0 ("disabled index (col)")) -> (element=w1160:string[])  [unwired: 1 in]
        n550 = Index Array(array=w1155, index (dim 0)=w1131, index (dim 2)=0 ("disabled index (row)")) -> (element=w1168:string[])  [unwired: 1 in]
        n551 = Array To Spreadsheet String(delimiter (Tab)=";", array=w1160, 3:"%s" ("format string")) -> (spreadsheet string=w1150:string)
        n552 = Search 1D Array(1D array=w1168, element="Command") -> (index of element=w1157:i32)  [unwired: 1 in]
        n553 = Match Pattern(string=w1150, regular expression=";;") -> (before substring=w1152:string)  [unwired: 4 out]
        n554 = Index Array(array=w1155, index (dim 0)=w1131, index (dim 1)=w1157, index (dim 2)=1 ("disabled index (col)")) -> (element=w1171:string)
        n555 = Match Pattern(string=w1152, regular expression="\r\n") -> (before substring=w1161:string)  [unwired: 4 out]
        n556 = Format Into String(format string="%s%s;", w1171, w1161) -> (resulting string=w1170:string)  [unwired: 2 in, 1 out]
        n557 = Array To Spreadsheet String(delimiter (Tab)=",", array=w1160, 3:"%s" ("format string")) -> (spreadsheet string=w1148:string)
        n558 = Search 1D Array(1D array=w1168, element="Telemetry") -> (index of element=w1154:i32)  [unwired: 1 in]
        n559 = call "NextState.vi"("Data"=w1170, "State"="Send Command", "Queue In"=w1145) -> ("Queue Out"=w1166:refnum<queue>)  [unwired: 7 in, 1 out]
        n560 = Match Pattern(string=w1148, regular expression=",,") -> (before substring=w1149:string)  [unwired: 4 out]
        n561 = Index Array(array=w1155, index (dim 0)=w1131, index (dim 1)=w1154, index (dim 2)=1 ("disabled index (col)")) -> (element=w1136:string)
        n562 = Match Pattern(string=w1149, regular expression="\r\n") -> (before substring=w1144:string)  [unwired: 4 out]
        n563 = property on="Parameter Type" class="Ring (strict)"() -> ("Strings []"=w1138:string[])  [unwired: 2 in, 2 out]
        n564 = call "NextState.vi"("Data"=w1136, "State"="Request Telemetry", "Queue In"=w1166) -> ("Queue Out"=w1165:refnum<queue>)  [unwired: 7 in, 1 out]
        n565 = Index Array(array=w1138, index=w1131) -> (element=w1137:string)
        n566 = Format Into String(format string="Uploaded %s parameters.", w1137) -> (resulting string=w1139:string)  [unwired: 2 in, 1 out]
        n567 = call "NextState.vi"("Data"=w1144, "State"="Verify Upload", "Queue In"=w1165) -> ("Queue Out"=w1143:refnum<queue>)  [unwired: 7 in, 1 out]
        n568 = call "NextState.vi"("State"="Update Parameter", "Queue In"=w1143) -> ("Queue Out"=w1142:refnum<queue>)  [unwired: 8 in, 1 out]
        n569 = call "NextState.vi"("Data"=w1139, "State"="Status", "Queue In"=w1142) -> ("Queue Out"=w1135:refnum<queue>)  [unwired: 7 in, 1 out]
        n570 = call "NextState.vi"("Data"=w1131, "State"="File Next", "Queue In"=w1135) -> ()  [unwired: 7 in, 2 out]
      }
      frame "File Save" {
        n571 = call "File Dialog2"("prompt"="Save AeroQuad Config File", "pattern (all files)"="*.aq", "pattern label"="AeroQuad Config") -> ("selected path"=w1181:path, "cancelled"=w1182:bool)  [unwired: 9 in, 2 out]
        n572 = case shown="False" w1182 {
          tunnel: w1186 -> [w1192 _]
          tunnel: w1181 -> [w1187 _]
          frame False {
            n573 = Unbundle By Name(w1192) -> ("ParameterName"=w1193:string[], "Parameters"=w1194:string[][][])
            n574 = property on="Parameter Type" class="Ring (strict)"() -> ("NumItems"=w1195:u32)  [unwired: 2 in, 2 out]
            n575 = call <vilib>:"Open Config Data.vi"("configuration file path"=w1187) -> ("error out"=w1191:errorcluster, "refnum"=w1188:T1)  [unwired: 8 in, 1 out]
            n576 = for {
              N: w1195 -> [_]
              tunnel: w1194 -> [w1205]
              tunnel: w1193 -> [w1200] mode=indexing
              shift-right: [w1198] -> w1190
              shift-left: w1191 -> [w1199]
              tunnel: [w1197] -> w1189
              tunnel: w1188 -> [w1196]
              i -> [w1204]
              n577 = Index Array(array=w1205, index (dim 0) #1=w1204, index (dim 0) #2=w1204, index (dim 2) #2=0 ("disabled index (col)")) -> (element #1=w1201:string[][], element #2=w1202:string[])  [unwired: 3 in]
              n578 = for {
                tunnel: w1202 -> [w1212] mode=indexing
                tunnel: w1201 -> [w1211] mode=indexing
                tunnel: w1200 -> [w1210]
                shift-right: [w1208] -> w1198
                shift-left: w1199 -> [w1209]
                tunnel: [w1207] -> w1197
                tunnel: w1196 -> [w1206]
                n579 = case shown="Default" w1212 {
                  tunnel: w1211 -> [w1219 _]
                  tunnel: w1210 -> [w1220 _]
                  tunnel: w1209 -> [w1216 w1222]
                  tunnel: [w1215 w1222] -> w1208
                  tunnel: [w1214 w1221] -> w1207
                  tunnel: w1206 -> [w1213 w1221]
                  frame Default {
                    n580 = Index Array(array=w1219) -> (element #1=w1218:string, element #2=w1217:string)  [unwired: 2 in]
                    n581 = call-poly <vilib>:"Write Key.vi"("section"=w1220, "error in (no error)"=w1216, "value"=w1217, "key"=w1218, "refnum"=w1213) -> ("error out"=w1215:errorcluster, "refnum out"=w1214:T1)  [unwired: 4 in, 1 out]
                  }
                  frame "Command", "Telemetry" {
                  }
                }
              }
            }
            n582 = call <vilib>:"Close Config Data.vi"("error in (no error)"=w1190, "refnum"=w1189) -> ()  [unwired: 8 in, 2 out]
          }
          frame True {
          }
        }
      }
      frame "--- Calibrations ---" {
      }
      frame "Store Calibration" {
        n583 = Unbundle By Name(w1237) -> ("IniPath"=w1226:path, "ConfigRef"=w1239:T1)
        n584 = Variant To Data(Variant=w1241, type=w1240) -> (data=w1235:string)  [unwired: 1 in, 1 out]
        n585 = Match Pattern(string=w1235, regular expression=";") -> (before substring=w1233:string, match substring=w1232:string, after substring=w1230:string)  [unwired: 1 in, 1 out]
        n586 = Concatenate Strings(w1233, w1232) -> (w1231:string)
        n587 = call-poly <vilib>:"Write Key.vi"("section"="Calibrations", "value"=w1230, "key"=w1231, "refnum"=w1239) -> ("error out"=w1228:errorcluster, "refnum out"=w1229:T1)  [unwired: 5 in, 1 out]
        n588 = call <vilib>:"Close Config Data.vi"("error in (no error)"=w1228, "refnum"=w1229) -> ("error out"=w1227:errorcluster)  [unwired: 8 in, 1 out]
        n589 = call <vilib>:"Open Config Data.vi"("error in (no error)"=w1227, "configuration file path"=w1226) -> ("error out"=w1225:errorcluster, "refnum"=w1224:T1)  [unwired: 7 in, 1 out]
        n590 = Bundle By Name(cluster=w1237, "ConfigRef"=w1224, "Error"=w1225) -> (w1236:T2)
      }
      frame "Recall Calibrations" {
        n591 = Variant To Data(Variant=w1253, type=w1252) -> (data=w1251:string)  [unwired: 1 in, 1 out]
        n592 = Unbundle By Name(w1250) -> ("ConfigRef"=w1249:T1)
        n593 = call "NextState.vi"("Data"="Recalling calibrations..." ("State"), "State"="Status", "Queue In"=w1247) -> ("Queue Out"=w1246:refnum<queue>)  [unwired: 7 in, 1 out]
        n594 = case shown="\"All\"" w1251 {
          selector: w1251 -> [w1255 _]
          tunnel: w1249 -> [w1266 w1300]
          tunnel: w1246 -> [w1256 w1294]
          tunnel: [w1257 w1297] -> w1242
          tunnel: [w1254 w1292] -> w1243
          frame Default {
            w1260 = "Calibrations" ("section")
            n595 = call-poly <vilib>:"Read Key.vi"("section"="Initial Setup", "key"=w1255, "refnum"=w1266) -> ("value"=w1263:string, "refnum out"=w1264:T1)  [unwired: 5 in, 2 out]
            n596 = call <vilib>:"Get Key Names.vi"("section"=w1260, "refnum"=w1264) -> ("key names"=w1262:string[], "refnum out"=w1261:T1)  [unwired: 6 in, 2 out]
            n597 = for {
              tunnel: w1263 -> [w1277]
              tunnel: w1262 -> [w1275] mode=indexing
              tunnel: w1261 -> [w1274]
              tunnel: [w1273] -> w1259 mode=indexing
              tunnel: w1260 -> [w1272]
              tunnel: w1256 -> [w1271]
              n598 = String Subset(string=w1275, length (rest)=1 ("length (rest)")) -> (substring=w1278:string)  [unwired: 1 in]
              n599 = Equal?(x=w1278, y=w1277) -> (x = y?=w1276:bool)
              n600 = case shown="True" w1276 {
                selector: w1276 -> [w1280 w1291]
                tunnel: w1275 -> [_ w1288]
                tunnel: w1274 -> [_ w1290]
                tunnel: [w1280 w1291] -> w1273
                tunnel: w1272 -> [_ w1289]
                tunnel: w1271 -> [_ w1286]
                frame False {
                }
                frame True {
                  n601 = call-poly <vilib>:"Read Key.vi"("section"=w1289, "key"=w1288, "refnum"=w1290) -> ("value"=w1287:string)  [unwired: 5 in, 3 out]
                  n602 = Concatenate Strings(w1288, w1287) -> (w1284:string)
                  n603 = call "NextState.vi"("Data"=w1284, "State"="Send Command", "Queue In"=w1286) -> ("Queue Out"=w1282:refnum<queue>)  [unwired: 7 in, 1 out]
                  n604 = call "NextState.vi"("Data"=100, "State"="Delay", "Queue In"=w1282) -> ()  [unwired: 7 in, 2 out]
                }
              }
            }
            n605 = Or Array Elements(Boolean array=w1259) -> (logical OR=w1258:bool)
            n606 = case shown="True" w1258 {
              tunnel: w1256 -> [w1267 w1270]
              tunnel: [w1267 w1270] -> w1257
              tunnel: w1255 -> [_ _]
              tunnel: ["No calibrations found." ("State") " Calibration Recalled" ("State")] -> w1254
              frame False {
              }
              frame True {
              }
            }
          }
          frame "All" {
            w1298 = "Calibrations" ("section")
            n607 = call <vilib>:"Get Key Names.vi"("section"=w1298, "refnum"=w1300) -> ("key names"=w1296:string[], "refnum out"=w1299:T1)  [unwired: 6 in, 2 out]
            n608 = for {
              tunnel: w1299 -> [w1320]
              tunnel: w1298 -> [w1319]
              tunnel: w1296 -> [w1311] mode=indexing
              tunnel: w1294 -> [w1318]
              tunnel: [w1312] -> w1293
              n609 = call-poly <vilib>:"Read Key.vi"("section"=w1319, "key"=w1311, "refnum"=w1320) -> ("value"=w1316:string)  [unwired: 5 in, 3 out]
              n610 = Match Pattern(string=w1311, regular expression="K") -> (offset past match=w1309:i32)  [unwired: 1 in, 3 out]
              n611 = Greater Or Equal To 0?(x=w1309) -> (x >= 0?=w1307:bool)
              n612 = Concatenate Strings(w1311, w1316) -> (w1315:string)
              n613 = call "NextState.vi"("Data"=w1315, "State"="Send Command", "Queue In"=w1318) -> ("Queue Out"=w1314:refnum<queue>)  [unwired: 7 in, 1 out]
              n614 = Select(t=1500, s=w1307, f=300) -> (s? t:f=w1305:i32)
              n615 = call "NextState.vi"("Data"=w1305, "State"="Delay", "Queue In"=w1314) -> ("Error Out"=w1312:errorcluster)  [unwired: 7 in, 1 out]
            }
            n616 = Array Size(array=w1296) -> (size(s)=w1295:i32)
            n617 = case shown="Default" w1295 {
              tunnel: w1294 -> [w1302 w1304]
              tunnel: [w1302 w1304] -> w1297
              tunnel: w1293 -> [_ _]
              tunnel: ["No calibrations found." ("State") "Calibrations Recalled" ("State")] -> w1292
              frame 0 {
              }
              frame Default {
              }
            }
          }
        }
        n618 = call "NextState.vi"("Data"=w1243, "State"="Cleanup Recall", "Queue In"=w1242) -> ()  [unwired: 7 in, 2 out]
      }
      frame "Cleanup Recall" {
        n619 = Get Queue Status(queue=w1326) -> (queue out=w1322:refnum<queue>, elements=w1325:cluster{"State":string, "Data":variant}[])  [unwired: 2 in, 6 out]
        n620 = for "Fix later - currently nothing happens" {
          tunnel: w1325 -> [w1351] mode=indexing
          tunnel: [w1347] -> w1324 mode=indexing
          n621 = Unbundle By Name(w1351) -> ("State"=w1349:string)
          n622 = Match Pattern(string=w1349, regular expression="Recall Calibrations") -> (offset past match=w1348:i32)  [unwired: 1 in, 3 out]
          n623 = Greater Or Equal To 0?(x=w1348) -> (x >= 0?=w1347:bool)
        }
        n624 = Or Array Elements(Boolean array=w1324) -> (logical OR=w1323:bool)
        n625 = case shown="False" w1323 {
          tunnel: w1322 -> [w1337 w1346]
          tunnel: w1321 -> [w1329 w1344]
          frame False {
            n626 = call "NextState.vi"("Data"="W", "State"="Send Command", "Queue In"=w1337) -> ("Queue Out"=w1336:refnum<queue>)  [unwired: 7 in, 1 out]
            n627 = call "NextState.vi"("Data"=6000, "State"="Delay", "Queue In"=w1336) -> ("Queue Out"=w1335:refnum<queue>)  [unwired: 7 in, 1 out]
            n628 = call "NextState.vi"("Data"=w1329, "State"="Status", "Queue In"=w1335) -> ("Queue Out"=w1334:refnum<queue>)  [unwired: 7 in, 1 out]
            n629 = call "NextState.vi"("State"="Unlock User Controls", "Queue In"=w1334) -> ("Queue Out"=w1332:refnum<queue>)  [unwired: 8 in, 1 out]
            n630 = call "NextState.vi"("State"="Load SubPanel", "Queue In"=w1332) -> ()  [unwired: 8 in, 2 out]
          }
          frame True {
            n631 = call "NextState.vi"("Data"=w1344, "State"="Status", "Queue In"=w1346) -> ("Queue Out"=w1342:refnum<queue>)  [unwired: 7 in, 1 out]
            n632 = call "NextState.vi"("Data"=6000, "State"="Delay", "Queue In"=w1342) -> ()  [unwired: 7 in, 2 out]
          }
        }
      }
    }
  }
  n633 = while {
    tunnel: w6 -> [w1355]
    tunnel: w3 -> [w1354]
    tunnel: [w1352] -> w5
    stop <- w1353 stop-if-true
    n634 = event shown="[1] Menu Selection (User)" {
      selector: w1355 -> [_ _ _ _ _]
      dyn-events: [_ _ _ _ _] -> w1352
      timeout: _ -> [_ _ _ _ _]
      tunnel: w1354 -> [w1357 w1365 w1394 w1402 w1404]
      tunnel: [_ w1363 TRUE _ _] -> w1353
      event Value Change {
        # "If a control 's value has changed,\nit's name will be called as a state.\nIt will not go to a state if it has a * in it's name."
        n635 = event-data() -> ("CtlRef"=w1360:refnum<vi>)  [unwired: 1 in]
        n636 = property class="Ctl"(reference=w1360) -> ("Label.Text"=w1356:string)  [unwired: 1 in, 2 out]
        n637 = Match Pattern(string=w1356, regular expression="*") -> (offset past match=w1358:i32)  [unwired: 1 in, 3 out]
        n638 = case shown="..0" w1358 {
          tunnel: w1357 -> [_ w1362]
          tunnel: w1356 -> [_ w1361]
          frame Default {
          }
          frame ..0 {
            n639 = call "NextState.vi"("State"=w1361, "Queue In"=w1362) -> ()  [unwired: 8 in, 2 out]
          }
        }
      }
      event Menu Selection (User) {
        n640 = event-data() -> ("ItemTag"=w1364:string)  [unwired: 1 in]
        n641 = case shown="\"Recall Calibrations:\"..\"Recall Calibrations:z\"" w1364 {
          selector: w1364 -> [w1370 w1374 w1389]
          tunnel: w1365 -> [w1367 w1375 w1380]
          tunnel: [TRUE _ _] -> w1363
          frame "Exit" {
            n642 = call "NextState.vi"("State"="Save Front Panel", "Queue In"=w1367) -> ("Queue Out"=w1368:refnum<queue>)  [unwired: 8 in, 1 out]
            n643 = call "NextState.vi"("State"=w1370, "Queue In"=w1368) -> ()  [unwired: 8 in, 2 out]
          }
          frame Default {
            n644 = Match Pattern(string=w1374, regular expression=":") -> (before substring=w1372:string, after substring=w1371:string)  [unwired: 1 in, 2 out]
            n645 = call "NextState.vi"("Data"=w1371, "State"=w1372, "Queue In"=w1375) -> ()  [unwired: 7 in, 2 out]
          }
          frame "Recall Calibrations:".."Recall Calibrations:z" {
            n646 = Flush Queue(queue=w1380) -> (queue out=w1379:refnum<queue>)  [unwired: 1 in, 2 out]
            n647 = call "NextState.vi"("State"="Clear Serial Comm" ("GUI State"), "Queue In"=w1379) -> ("Queue Out"=w1378:refnum<queue>)  [unwired: 8 in, 1 out]
            n648 = call "NextState.vi"("State"="Lock User Controls" ("GUI State"), "Queue In"=w1378) -> ("Queue Out"=w1376:refnum<queue>)  [unwired: 8 in, 1 out]
            n649 = Match Pattern(string=w1389, regular expression=":") -> (before substring=w1387:string, after substring=w1385:string)  [unwired: 1 in, 2 out]
            n650 = Spreadsheet String To Array(delimiter (Tab)=",", format string="%s", spreadsheet string=w1385, array type (2D Dbl)=string[] []) -> (array=w1382:string[])
            n651 = for {
              tunnel: w1387 -> [w1393]
              tunnel: w1382 -> [w1392] mode=indexing
              tunnel: [w1391] -> _
              tunnel: w1376 -> [w1390]
              n652 = call "NextState.vi"("Data"=w1392, "State"=w1393, "Queue In"=w1390) -> ("Queue Out"=w1391:refnum<queue>)  [unwired: 7 in, 1 out]
            }
          }
        }
      }
      event Panel Close? {
        n653 = event-data() -> ()  [unwired: 1 in, 1 out]
        n654 = call "NextState.vi"("State"="Save Front Panel", "Queue In"=w1394) -> ("Queue Out"=w1395:refnum<queue>)  [unwired: 8 in, 1 out]
        n655 = call "NextState.vi"("State"="Exit", "Queue In"=w1395) -> ()  [unwired: 8 in, 2 out]
        n656 = event-data("Discard?"=TRUE) -> ()  [unwired: 1 in, 1 out]
      }
      event "Parameter Check": Mouse Down {
        n657 = event-data() -> ()  [unwired: 1 in, 1 out]
        n658 = property on="Parameter Check" class="Tbl (strict)"() -> ("EditPos"=w1403:T5)  [unwired: 2 in, 2 out]
        n659 = Unbundle By Name(w1403) -> ("Row"=w1400:i32)
        n660 = call "NextState.vi"("Data"=w1400, "State"="Update Tool Tip", "Queue In"=w1402) -> ()  [unwired: 7 in, 2 out]
      }
      event Key Down {
        n661 = event-data() -> ("Char"=w1405:i16)  [unwired: 1 in]
        n662 = case shown="9" w1405 {
          tunnel: w1404 -> [w1407 _]
          frame 9 {
            n663 = call "NextState.vi"("State"="Next Parameter", "Queue In"=w1407) -> ()  [unwired: 8 in, 2 out]
          }
          frame Default {
          }
        }
      }
    }
  }
  n664 = Unregister For Events(event registration refnum=w5) -> ()  [unwired: 1 in, 1 out]
